vi "buildTestScenario.vi"(0 "TestScenarioFactory in":refnum<class "TestScenarioFactory.lvclass">, 5 "Log":refnum<class "ITestLog.lvclass">, 7 "Test Scenario":T1, 11 "error in (no error)":errorcluster) -> (4 "TestScenarioFactory out":refnum<class "TestScenarioFactory.lvclass">, 6 "ITestScenario.lvclass":refnum<class "ITestScenario.lvclass">, 15 "error out":errorcluster)   [LabVIEW 2015, in "TestScenarioFactory.lvclass"]
uses:
  TestScenarioFactory.lvclass
  Typedefs/TestScenarioTypes.ctl
  TestScenario/ITestScenario/ITestScenario.lvclass
  TestLog/ITestLog/ITestLog.lvclass
  TestScenario/Not Implemented Test/NotImplementedTest.lvclass
  TestScenario/Constant Analog Output Voltage Test/Constant Analog Output Voltage Test.lvclass
  TestScenarioFactory.lvclass/TestScenarioFactory.ctl
  TestScenario/Constant Current Output Test/Constant Current Output Test.lvclass
  TestScenario/Set DAC Test/Set ILC Test.lvclass
  ConfigureILCStrategy/ConfigureILCDCADAC1Strategy/ConfigureILCDCADAC1Strategy.lvclass
  ConfigureILCStrategy/ConfigureILCDCADAC2Strategy/ConfigureILCDCADAC2Strategy.lvclass
  ConfigureILCStrategy/ConfigureILCSSRStrategy/ConfigureILCSSRStrategy/ConfigureILCSSRStrategy.lvclass
  ConfigureILCStrategy/ConfigureILCDCAOutputStrategy/ConfigureILCDCAOutputStrategy.lvclass
  TestScenario/Verify ILC Test/Verify ILC Test.lvclass
  ReadILCStrategy/ReadILCDCAOutputStrategy/ReadILCDCAOutputStrategy.lvclass
  ConfigureILCStrategy/ConfigureILCDCAPressureStrategy/ConfigureILCDCAPressureStrategy.lvclass
  ReadILCStrategy/ReadILCDCAPowerFailStrategy/ReadILCDCAPowerFailStrategy.lvclass
  ReadILCStrategy/ReadILCDCAAmp1FailStrategy/ReadILCDCAAmp1FailStrategy.lvclass
  ReadILCStrategy/ReadILCDCAAmp2FailStrategy/ReadILCDCAAmp2FailStrategy.lvclass
  TestScenario/Test Pressure/Test Pressure.lvclass
  ConfigureILCStrategy/ConfigureILCDAC1Strategy/ConfigureILCDAC1Strategy.lvclass
  ReadILCStrategy/ReadILCDCAPressure1Strategy/ReadILCDCAPressure1Strategy.lvclass
  ConfigureILCStrategy/ConfigureILCDAC2Strategy/ConfigureILCDAC2Strategy.lvclass
  ReadILCStrategy/ReadILCDCAPressure2Strategy/ReadILCDCAPressure2Strategy.lvclass
  ConfigureILCStrategy/ConfigureILCDAC3Strategy/ConfigureILCDAC3Strategy.lvclass
  ReadILCStrategy/ReadILCDCAPressure3Strategy/ReadILCDCAPressure3Strategy.lvclass
  ConfigureILCStrategy/ConfigureILCDAC4Strategy/ConfigureILCDAC4Strategy.lvclass
  ReadILCStrategy/ReadILCDCAPressure4Strategy/ReadILCDCAPressure4Strategy.lvclass
  TestScenario/Current Linear Test/Current Linear Test.lvclass
  Typedefs/ILCBTTypedefs.lvlib
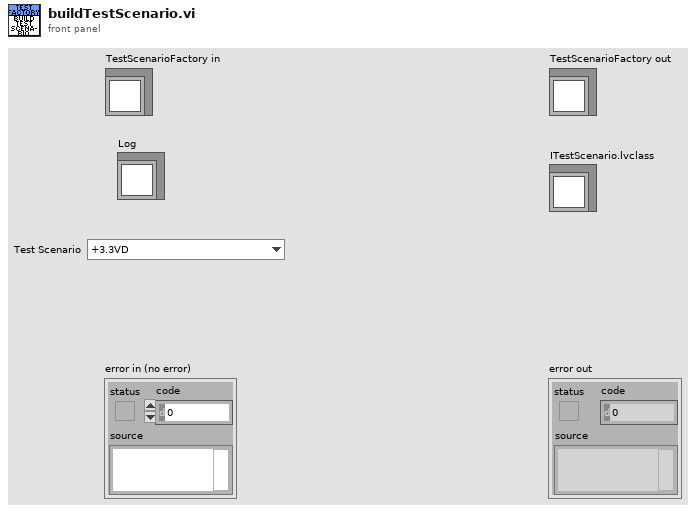
[diagram p1: front panel]
types:
  T1 = typedef "ILCBTTypedefs.lvlib/TestScenarioTypes.ctl" = enum16{"+3.3VD", "+5.1V", "+24V", "RELVALV1", "RELVALV2", "Verify DAC_A = -1.00A", "Verify DAC_A = -0.75A", "Verify DAC_A = -0.50A", "Verify DAC_A = -0.25A", "Verify DAC_A = 0.00A", "Verify DAC_A = 0.25A", "Verify DAC_A = 0.50A", "Verify DAC_A = 0.75A", "Verify DAC_A = 1.00A", "Verify DAC_B = -1.00A", "Verify DAC_B = -0.75A", "Verify DAC_B = -0.50A", "Verify DAC_B = -0.25A", "Verify DAC_B = 0.00A", "Verify DAC_B = 0.25A", "Verify DAC_B = 0.50A", "Verify DAC_B = 0.75A", "Verify DAC_B = 1.00A", "Set DAC_A = -1.00A", "Set DAC_A = -0.75A", "Set DAC_A = -0.50A", "Set DAC_A = -0.25A", "Set DAC_A = 0.00A", "Set DAC_A = 0.25A", "Set DAC_A = 0.50A", "Set DAC_A = 0.75A", "Set DAC_A = 1.00A", "Set DAC_B = -1.00A", "Set DAC_B = -0.75A", "Set DAC_B = -0.50A", "Set DAC_B = -0.25A", "Set DAC_B = 0.00A", "Set DAC_B = 0.25A", "Set DAC_B = 0.50A", "Set DAC_B = 0.75A", "Set DAC_B = 1.00A", "Set MTR_PWR = On", "Set MTR_PWR = Off", "Set OUTPUT = On", "Set OUTPUT = Off", "Verify OUTPUT = On", "Verify OUTPUT = Off", "Verify POWER = Ok", "Verify POWER = Fail", "Verify AMP1 = Ok", "Verify AMP1 = Fail", "Verify AMP2 = Ok", "Verify AMP2 = Fail", "P1 0%", "P1 25%", "P1 50%", "P1 75%", "P1 100%", "P2 0%", "P2 25%", "P2 50%", "P2 75%", "P2 100%", "P3 0%", "P3 25%", "P3 50%", "P3 75%", "P3 100%", "P4 0%", "P4 25%", "P4 50%", "P4 75%", "P4 100%", "DCA 1 Linearity", "DCA 2 Linearity"}
  T2 = typedef "ILCBTTypedefs.lvlib/Pressure Test.ctl" = cluster{"Command":u16, "Expected":u16, "Tolerance":u16}
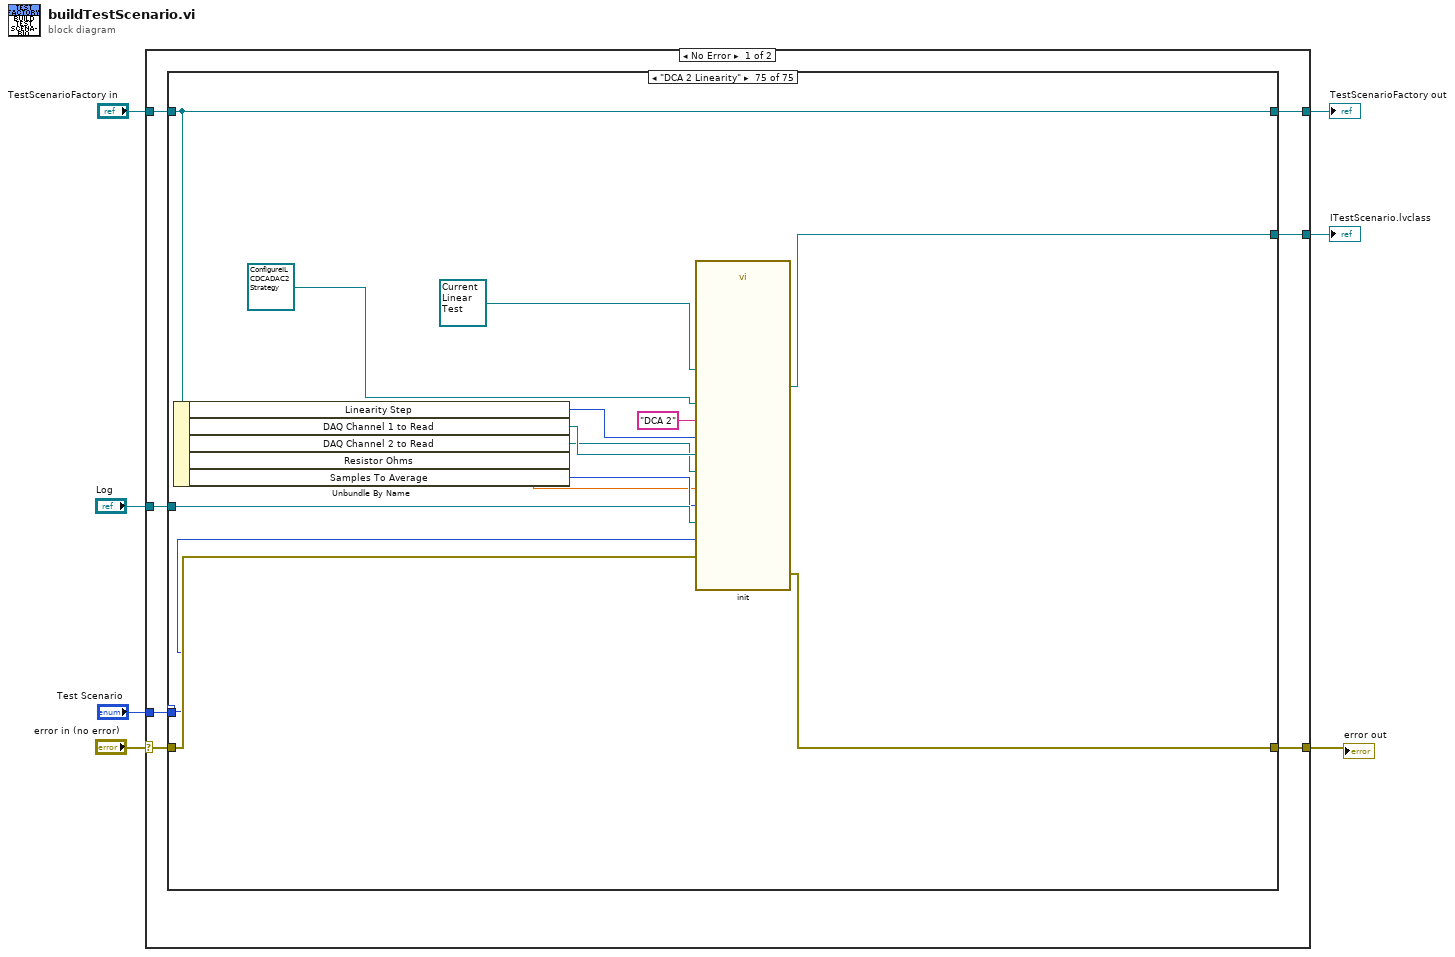
[diagram p0: block diagram]
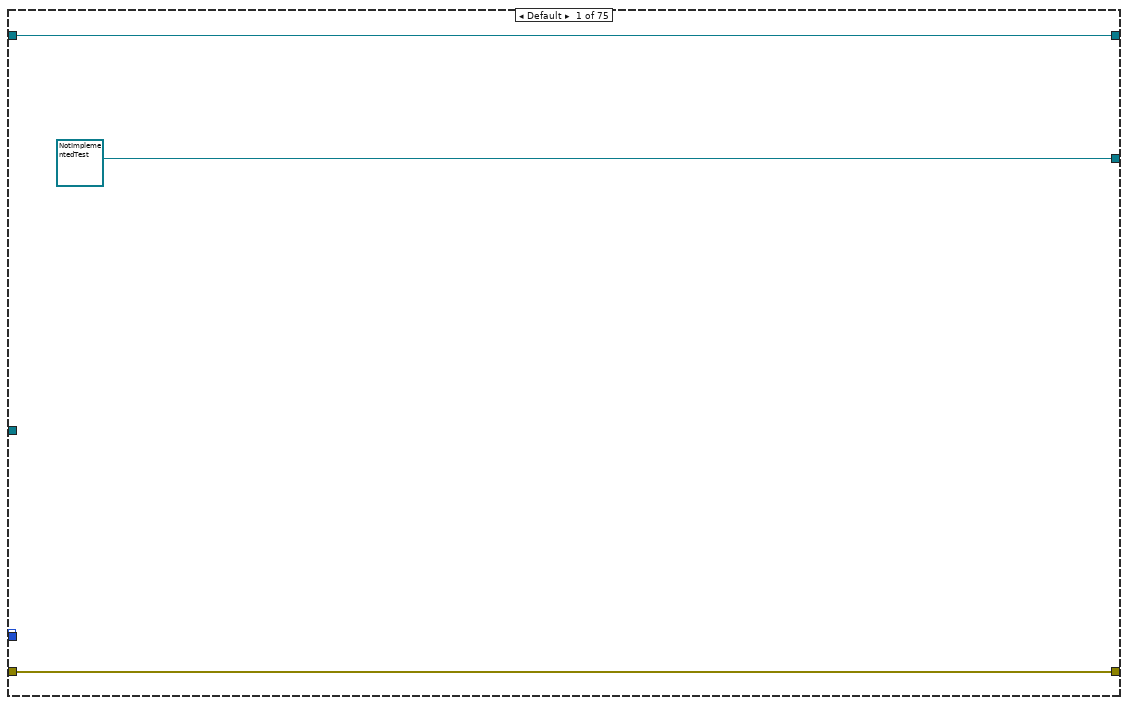
[diagram p2: hidden frame]
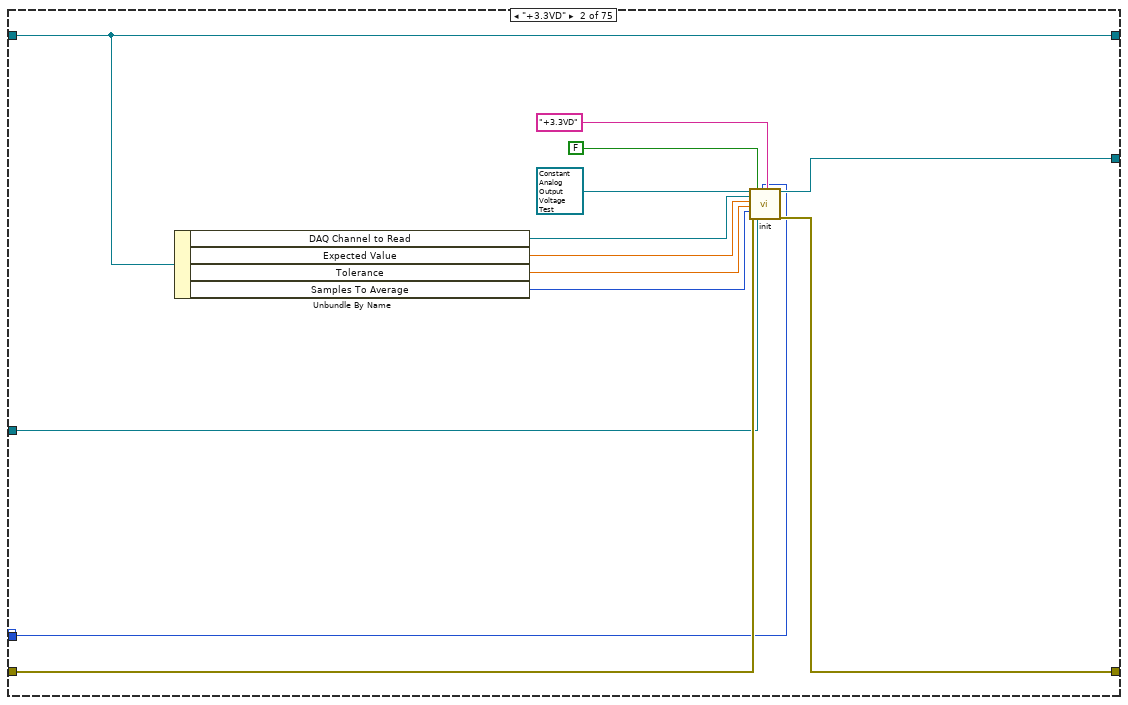
[diagram p3: hidden frame]
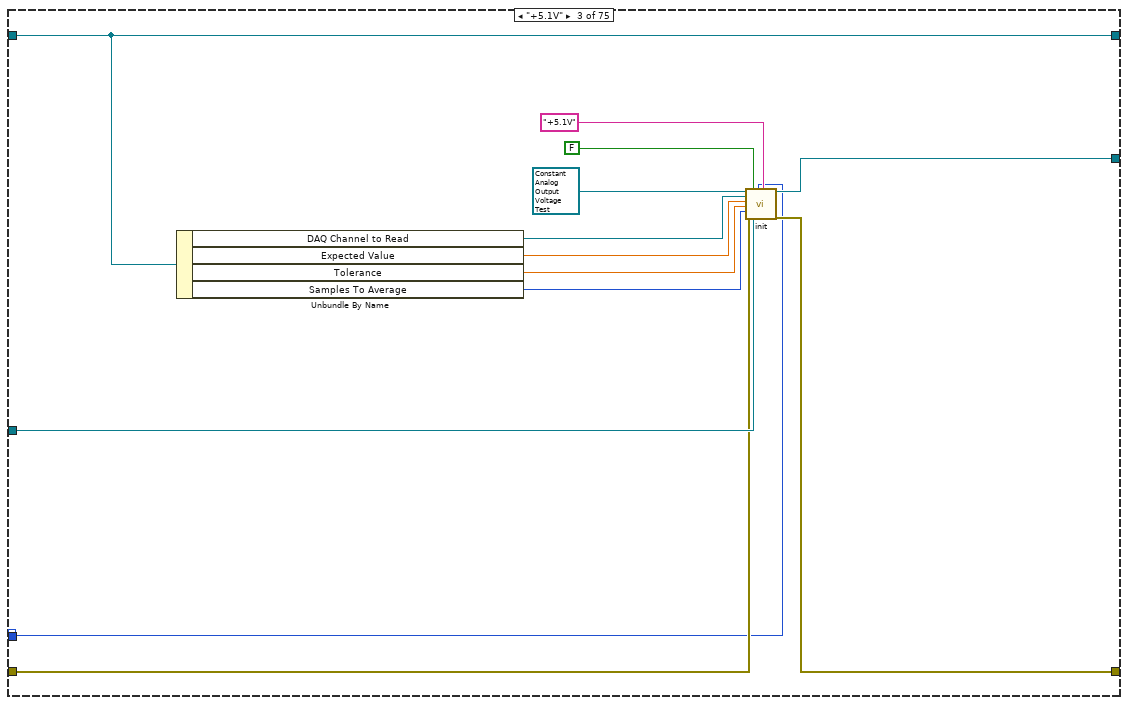
[diagram p4: hidden frame]
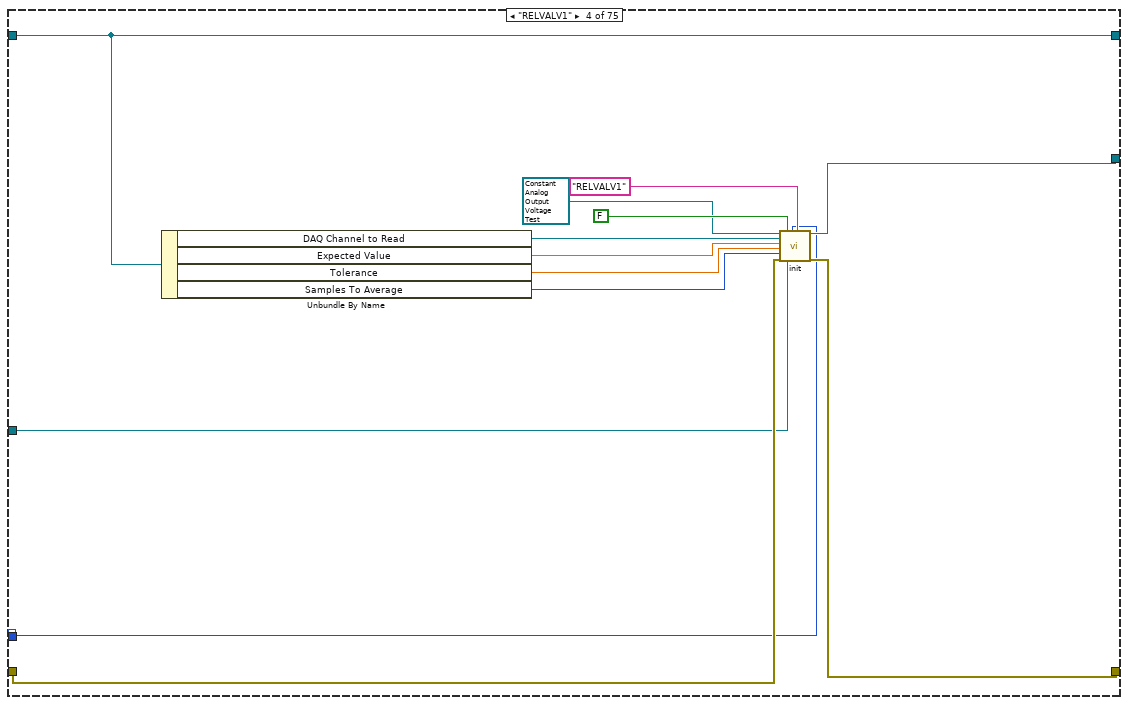
[diagram p5: hidden frame]
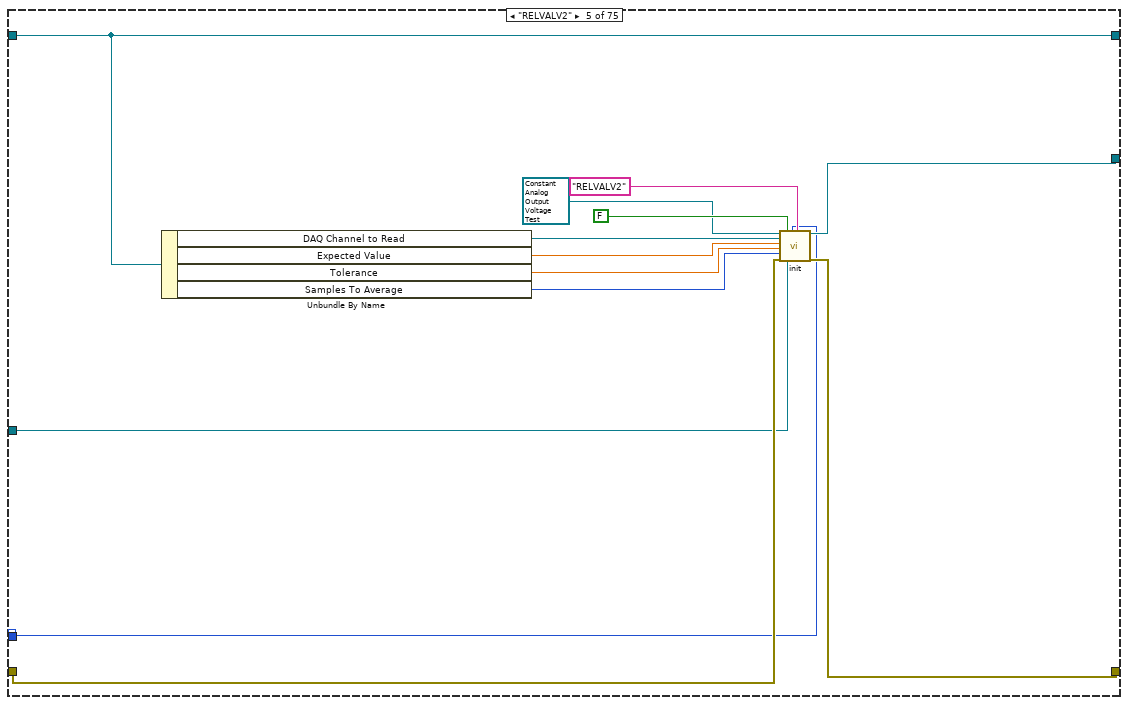
[diagram p6: hidden frame]
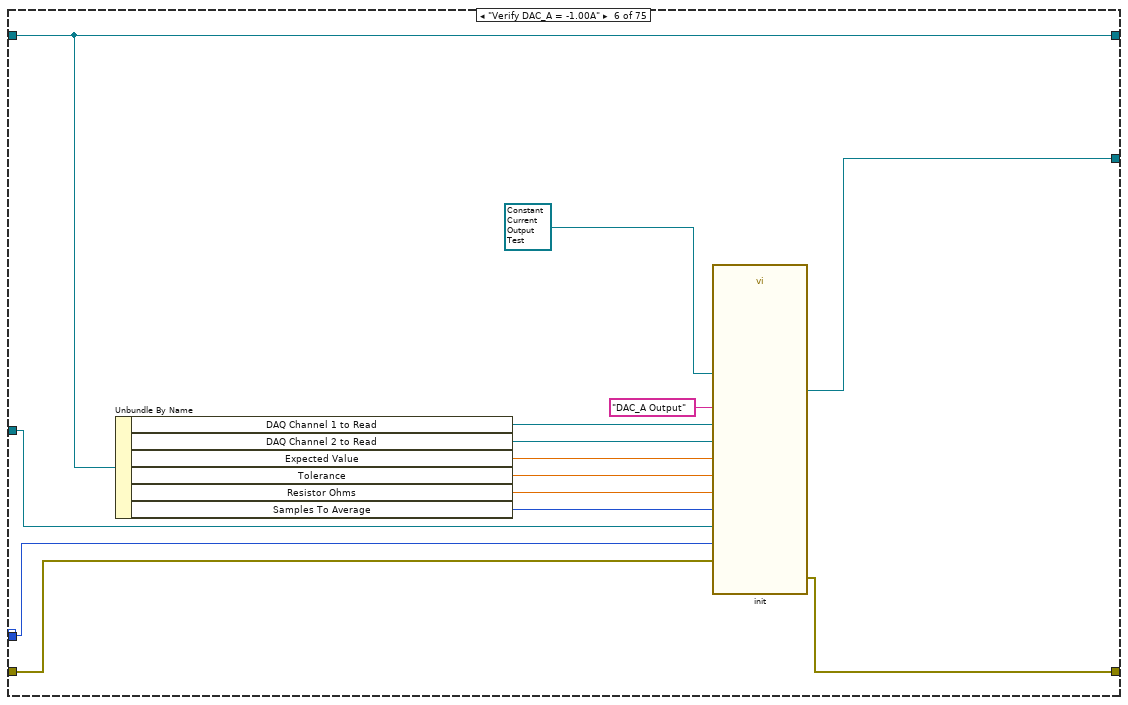
[diagram p7: hidden frame]
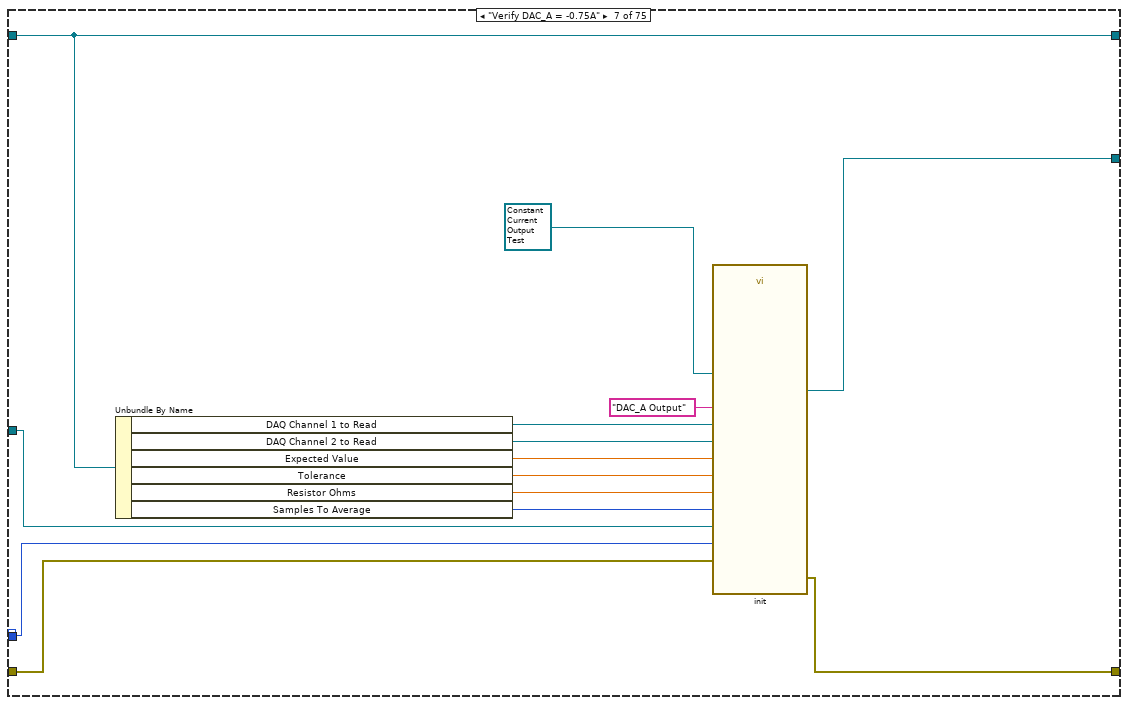
[diagram p8: hidden frame]
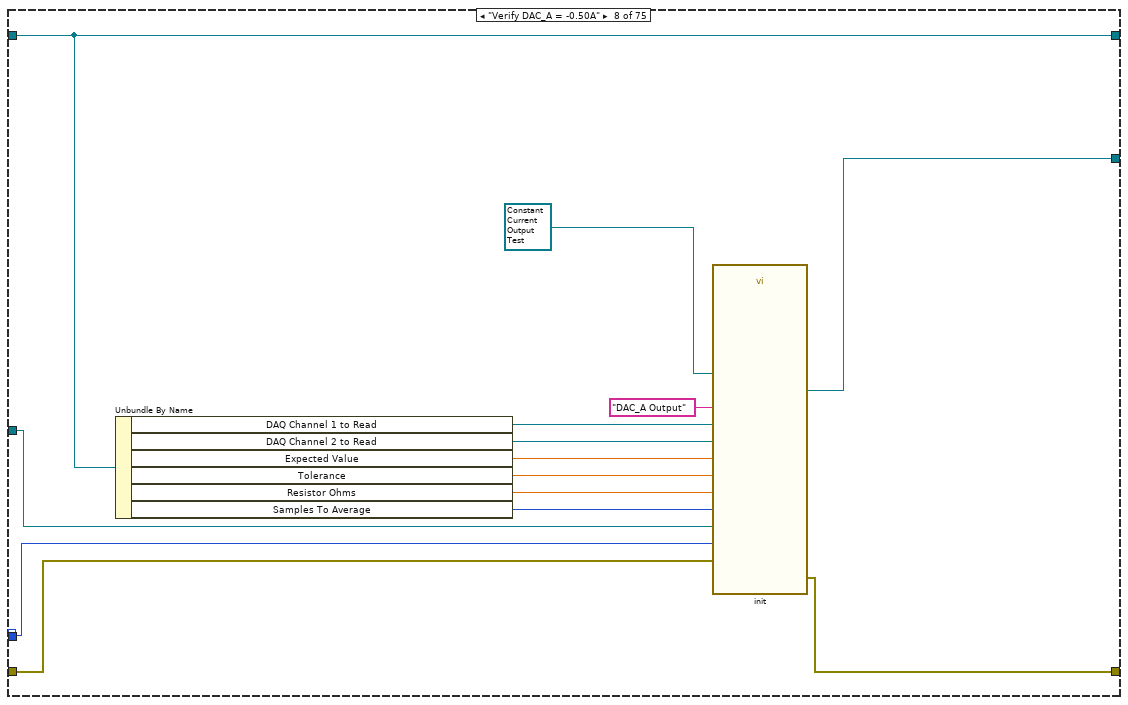
[diagram p9: hidden frame]
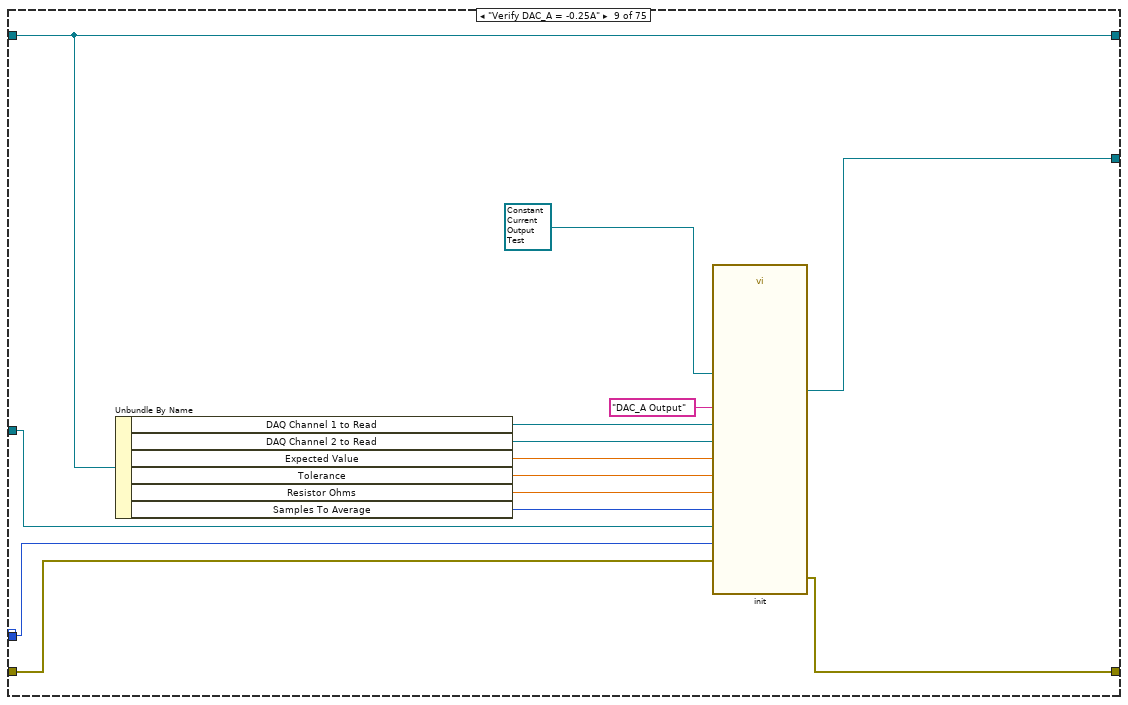
[diagram p10: hidden frame]
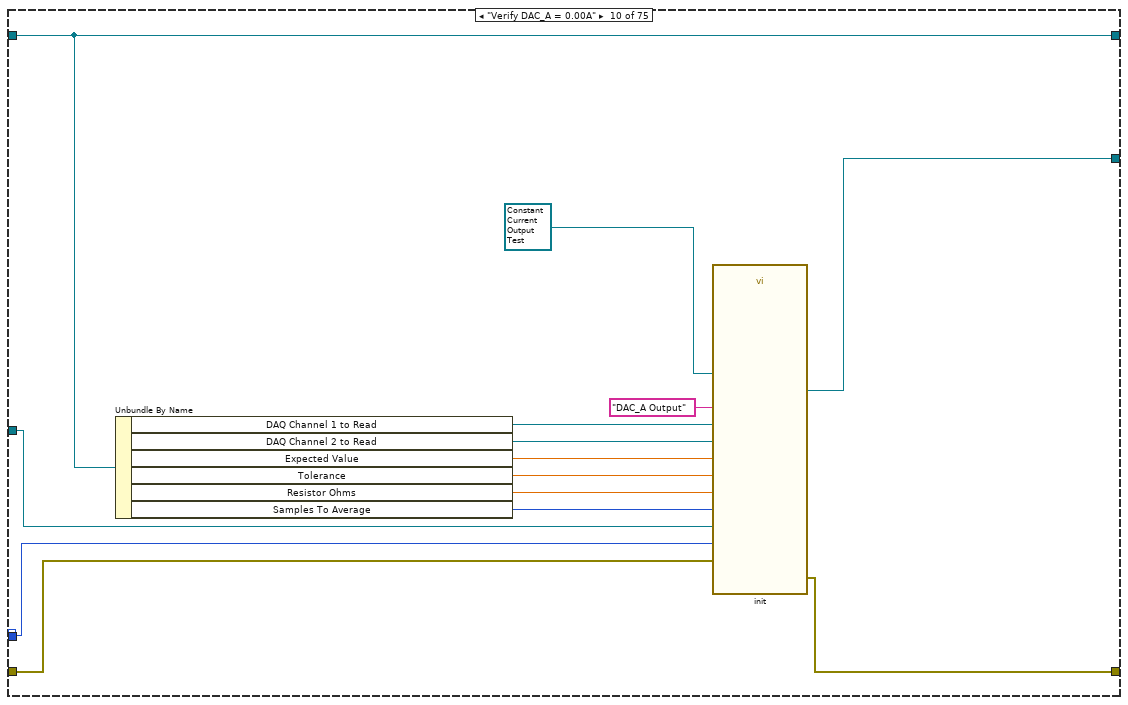
[diagram p11: hidden frame]
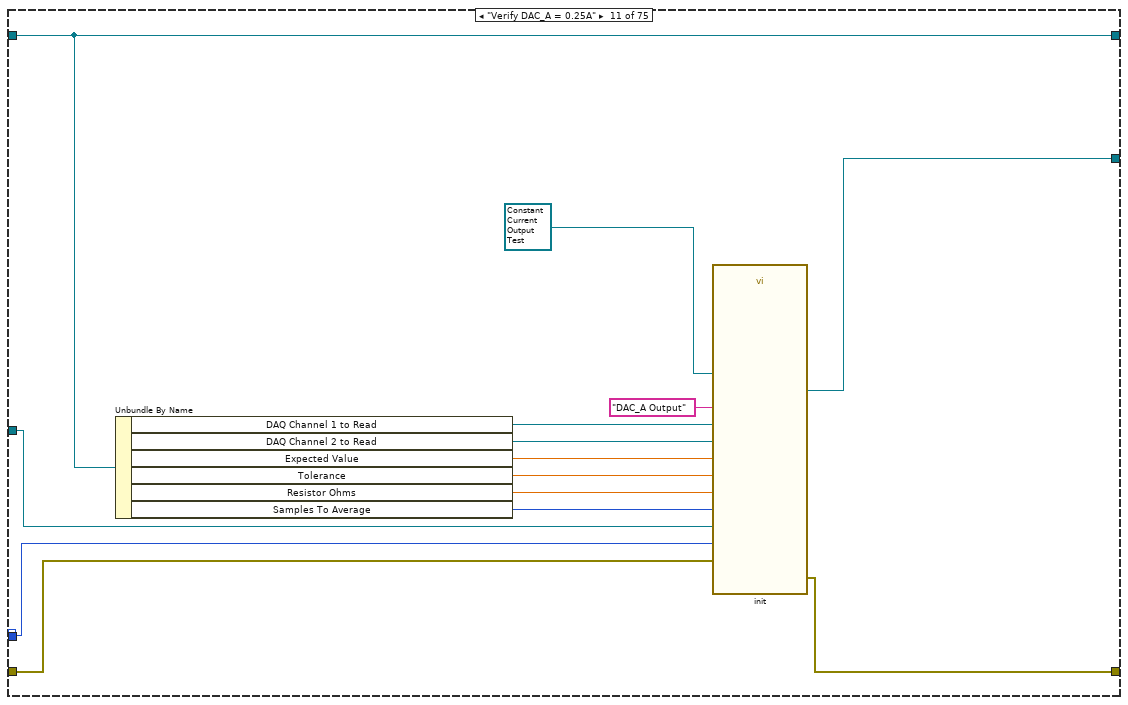
[diagram p12: hidden frame]
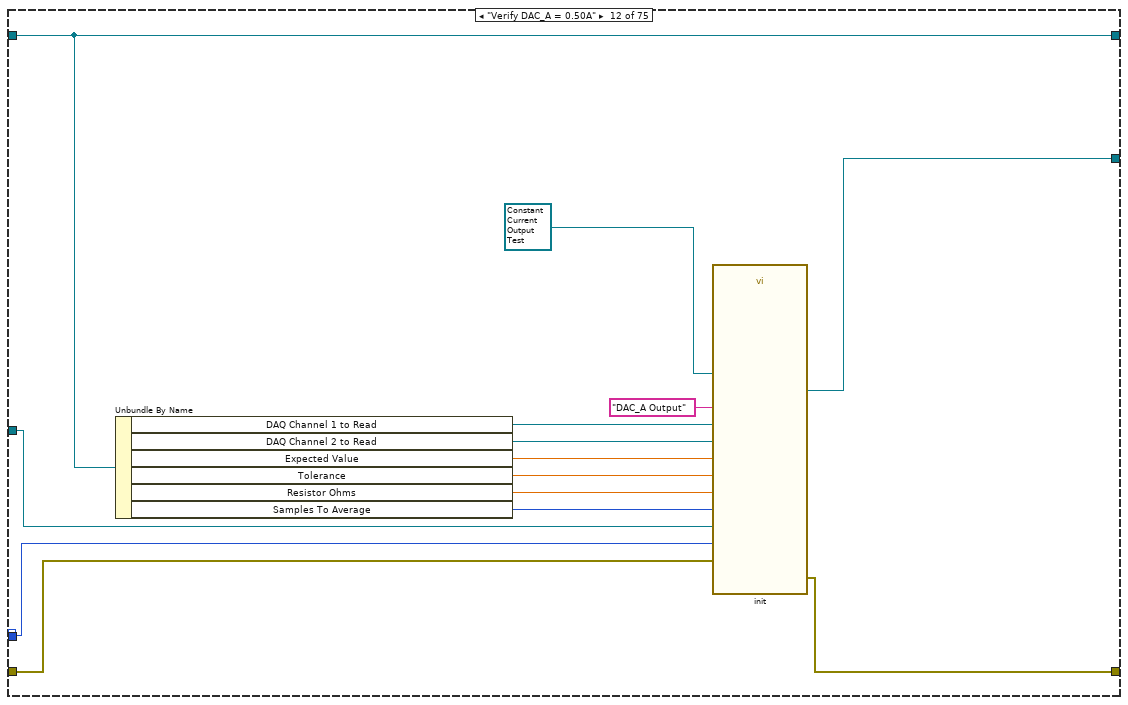
[diagram p13: hidden frame]
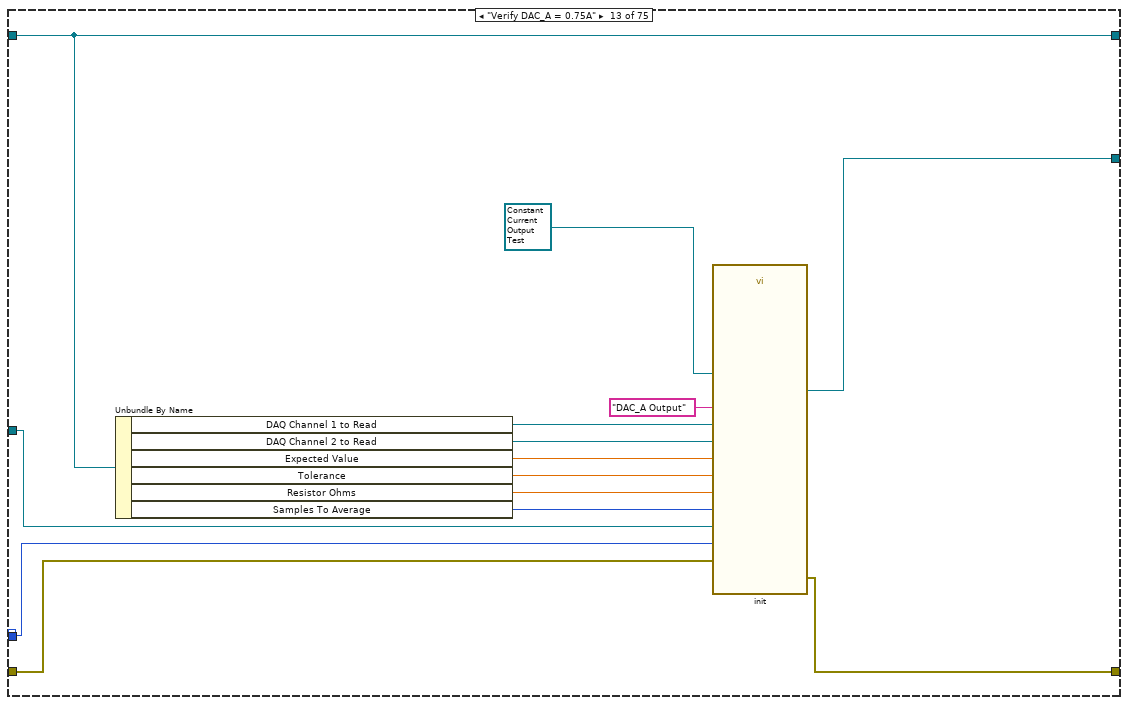
[diagram p14: hidden frame]
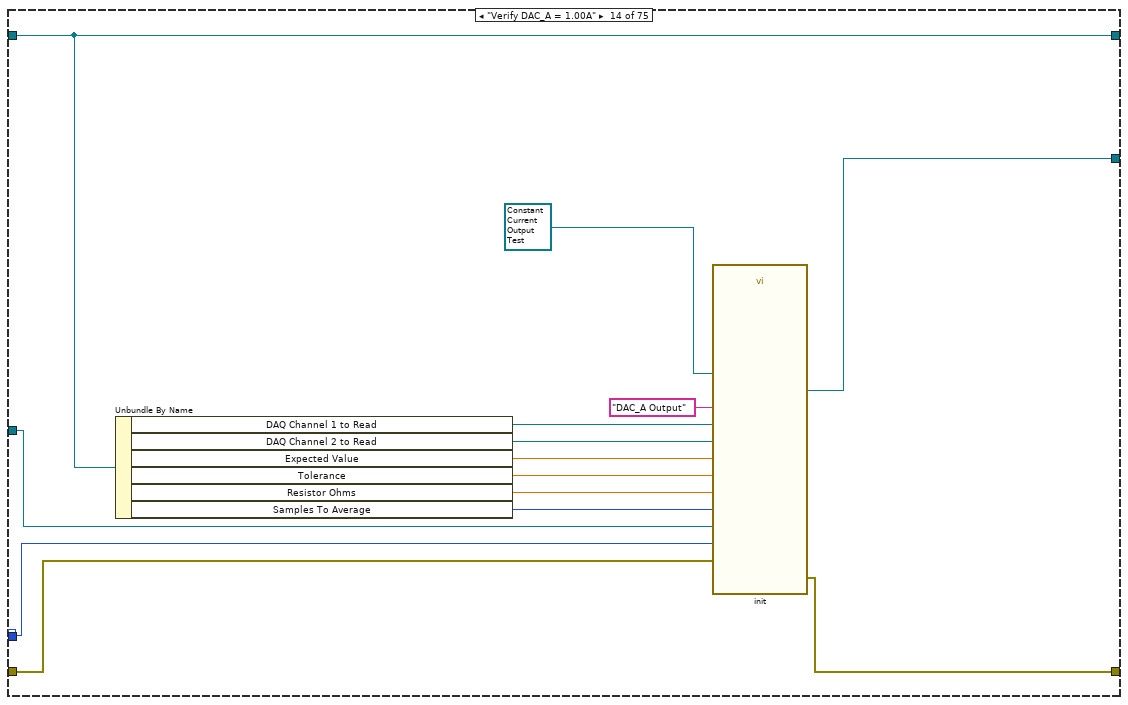
[diagram p15: hidden frame]
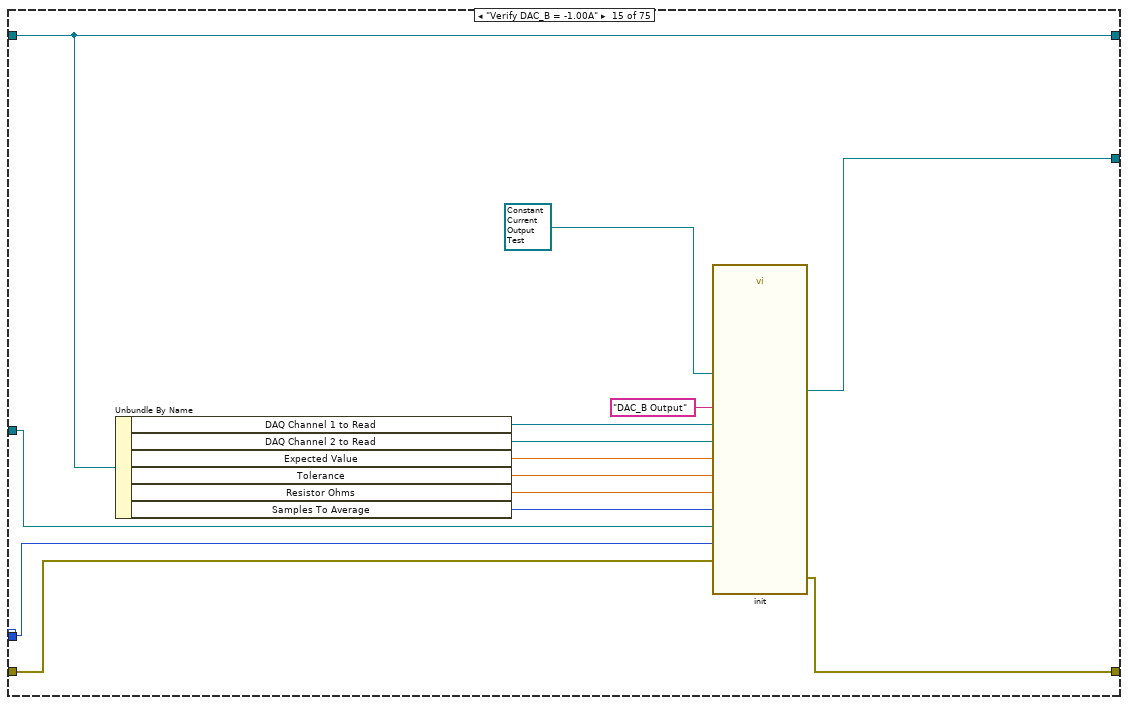
[diagram p16: hidden frame]
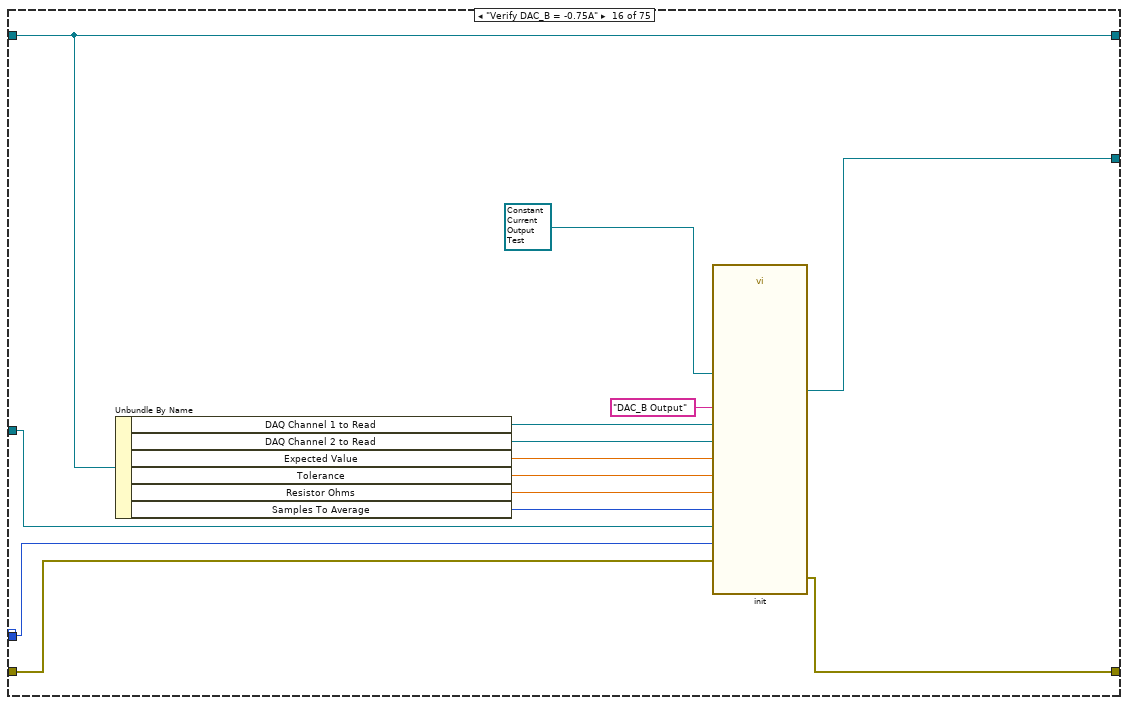
[diagram p17: hidden frame]
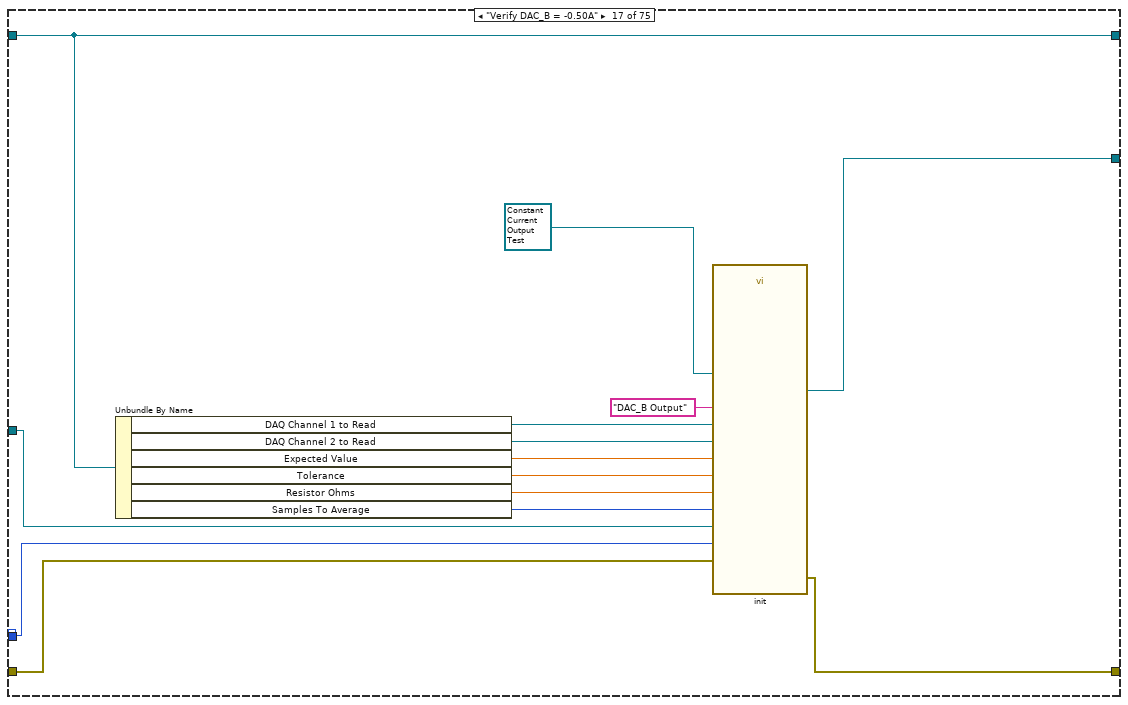
[diagram p18: hidden frame]
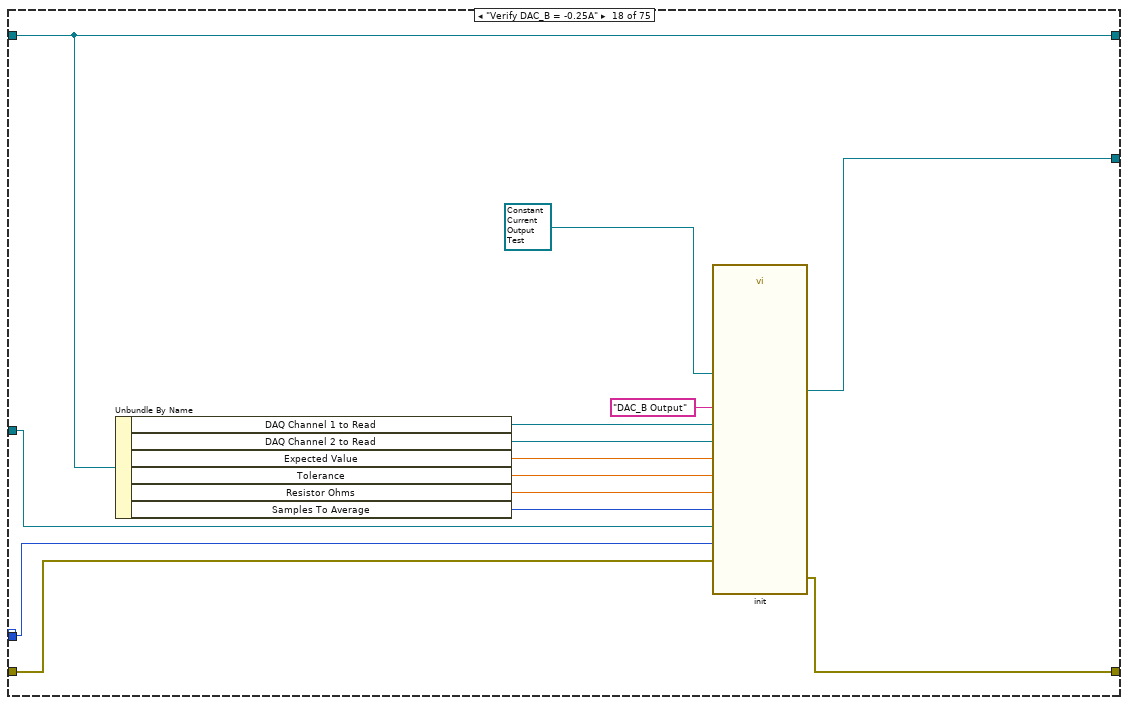
[diagram p19: hidden frame]
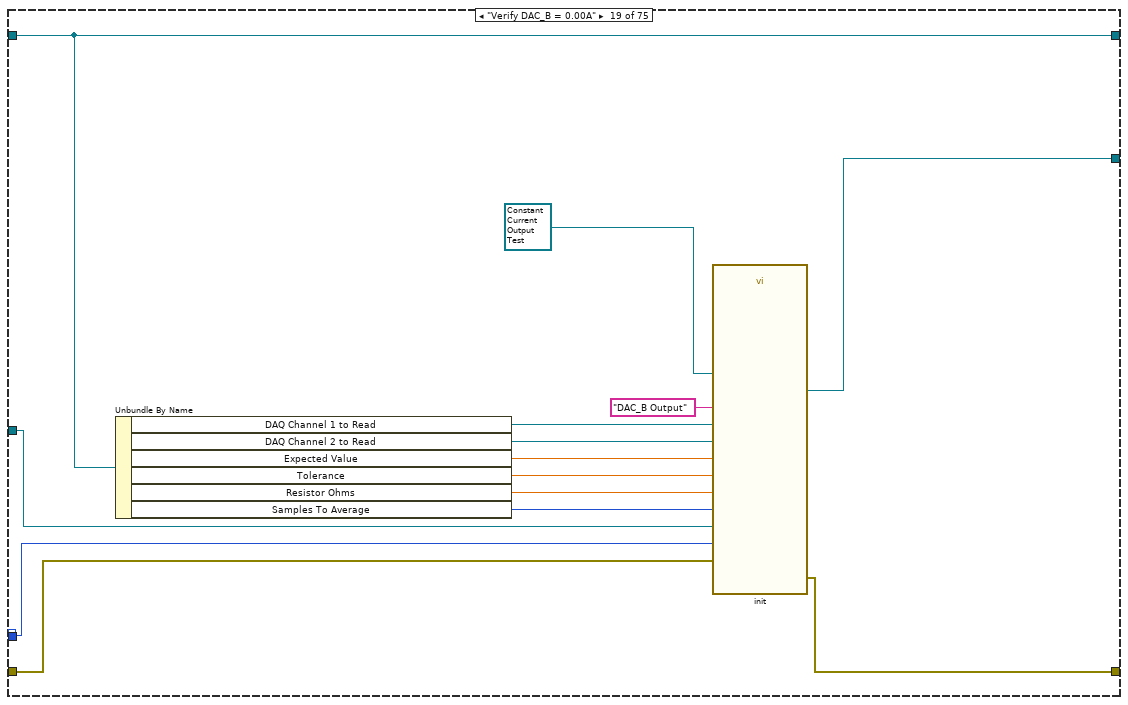
[diagram p20: hidden frame]
diagram:
  n1 = case shown="No Error" "error in (no error)" {
    selector: "error in (no error)" -> [w13 w948]
    tunnel: "Test Scenario" -> [w8 _]
    tunnel: "TestScenarioFactory in" -> [w14 w947]
    tunnel: [w12 w948] -> w3
    tunnel: [w9 w947] -> w5
    tunnel: "Log" -> [w10 _]
    tunnel: [w11 refnum<class "ITestScenario.lvclass"> refnum ("ITestScenario.lvclass")] -> w1
    frame No Error {
      n2 = case shown="\"DCA 2 Linearity\"" w8 {
        selector: w8 -> [_ w18 w31 w44 w57 w79 w93 w107 w121 w135 w149 w163 w177 w191 w205 w219 w233 w247 w261 w275 w289 w303 w317 w329 w339 w349 w359 w369 w379 w389 w399 w409 w419 w429 w439 w449 w459 w469 w479 w489 w499 w509 w519 w529 w539 w548 w560 w572 w584 w596 w608 w620 w632 w647 w661 w675 w689 w703 w717 w731 w745 w759 w773 w787 w801 w815 w829 w843 w857 w871 w885 w899 w913 w928 w942]
        tunnel: w14 -> [w17 w30 w34 w45 w58 w78 w92 w106 w120 w134 w148 w162 w176 w190 w204 w218 w232 w246 w260 w274 w288 w302 w316 w324 w334 w344 w354 w364 w374 w384 w394 w404 w415 w425 w435 w445 w455 w465 w475 w485 w495 w505 w515 w525 w535 w553 w565 w577 w589 w601 w613 w625 w637 w642 w656 w670 w684 w698 w714 w728 w742 w756 w770 w784 w798 w812 w826 w840 w854 w868 w882 w896 w910 w918 w933]
        tunnel: w13 -> [w16 w27 w35 w48 w61 w83 w97 w111 w125 w139 w153 w167 w181 w195 w209 w223 w237 w251 w265 w279 w293 w307 w321 w328 w338 w348 w358 w368 w378 w388 w398 w408 w418 w428 w438 w448 w458 w468 w478 w488 w498 w508 w518 w528 w538 w549 w561 w573 w585 w597 w609 w621 w633 w649 w663 w677 w691 w705 w719 w733 w747 w761 w775 w789 w803 w817 w831 w845 w859 w873 w887 w901 w915 w929 w943]
        tunnel: [w16 w19 w32 w49 w62 w82 w96 w110 w124 w138 w152 w166 w180 w194 w208 w222 w236 w250 w264 w278 w292 w306 w320 w327 w337 w347 w357 w367 w377 w387 w397 w407 w417 w427 w437 w447 w457 w467 w477 w487 w497 w507 w517 w527 w537 w550 w562 w574 w586 w598 w610 w622 w634 w648 w662 w676 w690 w704 w718 w732 w746 w760 w774 w788 w802 w816 w830 w844 w858 w872 w886 w900 w914 w927 w941] -> w12
        tunnel: [refnum<class "NotImplementedTest.lvclass"> refnum ("NotImplementedTest.lvclass") w28 w33 w46 w59 w81 w95 w109 w123 w137 w151 w165 w179 w193 w207 w221 w235 w249 w263 w277 w291 w305 w319 w331 w341 w351 w361 w371 w381 w391 w401 w411 w421 w431 w441 w451 w461 w471 w481 w491 w501 w511 w521 w531 w541 w551 w563 w575 w587 w599 w611 w623 w635 w650 w664 w678 w692 w706 w720 w734 w748 w762 w776 w790 w804 w818 w832 w846 w860 w874 w888 w902 w916 w930 w944] -> w11
        tunnel: w10 -> [_ w26 w36 w47 w60 w80 w94 w108 w122 w136 w150 w164 w178 w192 w206 w220 w234 w248 w262 w276 w290 w304 w318 w326 w336 w346 w356 w366 w376 w386 w396 w406 w416 w426 w436 w446 w456 w466 w476 w486 w496 w506 w516 w526 w536 w547 w559 w571 w583 w595 w607 w619 w631 w646 w660 w674 w688 w702 w716 w730 w744 w758 w772 w786 w800 w814 w828 w842 w856 w870 w884 w898 w912 w926 w940]
        tunnel: [w17 w30 w34 w45 w58 w78 w92 w106 w120 w134 w148 w162 w176 w190 w204 w218 w232 w246 w260 w274 w288 w302 w316 w324 w334 w344 w354 w364 w374 w384 w394 w404 w415 w425 w435 w445 w455 w465 w475 w485 w495 w505 w515 w525 w535 w553 w565 w577 w589 w601 w613 w625 w637 w642 w656 w670 w684 w698 w714 w728 w742 w756 w770 w784 w798 w812 w826 w840 w854 w868 w882 w896 w910 w918 w933] -> w9
        tunnel: w8 -> [_ _ _ _ _ _ _ _ _ _ _ _ _ _ _ _ _ _ _ _ _ _ _ _ _ _ _ _ _ _ _ _ _ _ _ _ _ _ _ _ _ _ _ _ _ _ _ _ _ _ _ _ _ _ _ _ _ _ _ _ _ _ _ _ _ _ _ _ _ _ _ _ _ _ _]
        frame Default {
        }
        frame "+3.3VD" {
          n3 = Unbundle By Name(w30) -> ("DAQ Channel to Read"=w22:refnum<k21>, "Expected Value"=w23:dbl, "Tolerance"=w24:dbl, "Samples To Average"=w25:i32)
          n4 = call "init.vi"("Constant Analog Output Voltage Test in"=refnum<class "Constant Analog Output Voltage Test.lvclass"> refnum ("Constant Analog Input Voltage Test.lvclass"), "DAQ Channel"=w22, "Expected Value"=w23, "Tolerance"=w24, "Samples To Average"=w25, "error in (no error)"=w27, "MustPass?"=FALSE, "Log"=w26, "Test Scenario"=w18, "Signal Name"="+3.3VD") -> ("Constant Analog Output Voltage Test  out"=w28:refnum<class "Constant Analog Output Voltage Test.lvclass">, "error out"=w19:errorcluster)  [unwired: 8 in]
        }
        frame "+5.1V" {
          n5 = Unbundle By Name(w34) -> ("DAQ Channel to Read"=w39:refnum<k21>, "Expected Value"=w40:dbl, "Tolerance"=w41:dbl, "Samples To Average"=w42:i32)
          n6 = call "init.vi"("Constant Analog Output Voltage Test in"=refnum<class "Constant Analog Output Voltage Test.lvclass"> refnum ("Constant Analog Input Voltage Test.lvclass"), "DAQ Channel"=w39, "Expected Value"=w40, "Tolerance"=w41, "Samples To Average"=w42, "error in (no error)"=w35, "MustPass?"=FALSE, "Log"=w36, "Test Scenario"=w31, "Signal Name"="+5.1V") -> ("Constant Analog Output Voltage Test  out"=w33:refnum<class "Constant Analog Output Voltage Test.lvclass">, "error out"=w32:errorcluster)  [unwired: 8 in]
        }
        frame "RELVALV1" {
          n7 = Unbundle By Name(w45) -> ("DAQ Channel to Read"=w54:refnum<k21>, "Expected Value"=w53:dbl, "Tolerance"=w52:dbl, "Samples To Average"=w51:i32)
          n8 = call "init.vi"("Constant Analog Output Voltage Test in"=refnum<class "Constant Analog Output Voltage Test.lvclass"> refnum ("Constant Analog Input Voltage Test.lvclass"), "DAQ Channel"=w54, "Expected Value"=w53, "Tolerance"=w52, "Samples To Average"=w51, "error in (no error)"=w48, "MustPass?"=FALSE, "Log"=w47, "Test Scenario"=w44, "Signal Name"="RELVALV1") -> ("Constant Analog Output Voltage Test  out"=w46:refnum<class "Constant Analog Output Voltage Test.lvclass">, "error out"=w49:errorcluster)  [unwired: 8 in]
        }
        frame "RELVALV2" {
          n9 = Unbundle By Name(w58) -> ("DAQ Channel to Read"=w67:refnum<k21>, "Expected Value"=w66:dbl, "Tolerance"=w65:dbl, "Samples To Average"=w64:i32)
          n10 = call "init.vi"("Constant Analog Output Voltage Test in"=refnum<class "Constant Analog Output Voltage Test.lvclass"> refnum ("Constant Analog Input Voltage Test.lvclass"), "DAQ Channel"=w67, "Expected Value"=w66, "Tolerance"=w65, "Samples To Average"=w64, "error in (no error)"=w61, "MustPass?"=FALSE, "Log"=w60, "Test Scenario"=w57, "Signal Name"="RELVALV2") -> ("Constant Analog Output Voltage Test  out"=w59:refnum<class "Constant Analog Output Voltage Test.lvclass">, "error out"=w62:errorcluster)  [unwired: 8 in]
        }
        frame "Verify DAC_A = -1.00A" {
          n11 = Unbundle By Name(w78) -> ("DAQ Channel 1 to Read"=w72:refnum<k21>, "DAQ Channel 2 to Read"=w73:refnum<k21>, "Expected Value"=w74:dbl, "Tolerance"=w75:dbl, "Resistor Ohms"=w76:dbl, "Samples To Average"=w77:i32)
          n12 = call "init.vi"("Constant Analog Output Voltage Test in"=refnum<class "Constant Current Output Test.lvclass"> refnum ("Constant Current Output Test.lvclass"), "DAQ Channel 1"=w72, "Expected Value"=w74, "Tolerance"=w75, "Samples To Average"=w77, "error in (no error)"=w83, "DAQ Channel 2"=w73, "Log"=w80, "Test Scenario"=w79, "Resistance"=w76, "Signal Name"="DAC_A Output") -> ("Constant Analog Output Voltage Test  out"=w81:refnum<class "Constant Current Output Test.lvclass">, "error out"=w82:errorcluster)  [unwired: 7 in]
        }
        frame "Verify DAC_A = -0.75A" {
          n13 = Unbundle By Name(w92) -> ("DAQ Channel 1 to Read"=w86:refnum<k21>, "DAQ Channel 2 to Read"=w87:refnum<k21>, "Expected Value"=w88:dbl, "Tolerance"=w89:dbl, "Resistor Ohms"=w90:dbl, "Samples To Average"=w91:i32)
          n14 = call "init.vi"("Constant Analog Output Voltage Test in"=refnum<class "Constant Current Output Test.lvclass"> refnum ("Constant Current Output Test.lvclass"), "DAQ Channel 1"=w86, "Expected Value"=w88, "Tolerance"=w89, "Samples To Average"=w91, "error in (no error)"=w97, "DAQ Channel 2"=w87, "Log"=w94, "Test Scenario"=w93, "Resistance"=w90, "Signal Name"="DAC_A Output") -> ("Constant Analog Output Voltage Test  out"=w95:refnum<class "Constant Current Output Test.lvclass">, "error out"=w96:errorcluster)  [unwired: 7 in]
        }
        frame "Verify DAC_A = -0.50A" {
          n15 = Unbundle By Name(w106) -> ("DAQ Channel 1 to Read"=w100:refnum<k21>, "DAQ Channel 2 to Read"=w101:refnum<k21>, "Expected Value"=w102:dbl, "Tolerance"=w103:dbl, "Resistor Ohms"=w104:dbl, "Samples To Average"=w105:i32)
          n16 = call "init.vi"("Constant Analog Output Voltage Test in"=refnum<class "Constant Current Output Test.lvclass"> refnum ("Constant Current Output Test.lvclass"), "DAQ Channel 1"=w100, "Expected Value"=w102, "Tolerance"=w103, "Samples To Average"=w105, "error in (no error)"=w111, "DAQ Channel 2"=w101, "Log"=w108, "Test Scenario"=w107, "Resistance"=w104, "Signal Name"="DAC_A Output") -> ("Constant Analog Output Voltage Test  out"=w109:refnum<class "Constant Current Output Test.lvclass">, "error out"=w110:errorcluster)  [unwired: 7 in]
        }
        frame "Verify DAC_A = -0.25A" {
          n17 = Unbundle By Name(w120) -> ("DAQ Channel 1 to Read"=w114:refnum<k21>, "DAQ Channel 2 to Read"=w115:refnum<k21>, "Expected Value"=w116:dbl, "Tolerance"=w117:dbl, "Resistor Ohms"=w118:dbl, "Samples To Average"=w119:i32)
          n18 = call "init.vi"("Constant Analog Output Voltage Test in"=refnum<class "Constant Current Output Test.lvclass"> refnum ("Constant Current Output Test.lvclass"), "DAQ Channel 1"=w114, "Expected Value"=w116, "Tolerance"=w117, "Samples To Average"=w119, "error in (no error)"=w125, "DAQ Channel 2"=w115, "Log"=w122, "Test Scenario"=w121, "Resistance"=w118, "Signal Name"="DAC_A Output") -> ("Constant Analog Output Voltage Test  out"=w123:refnum<class "Constant Current Output Test.lvclass">, "error out"=w124:errorcluster)  [unwired: 7 in]
        }
        frame "Verify DAC_A = 0.00A" {
          n19 = Unbundle By Name(w134) -> ("DAQ Channel 1 to Read"=w128:refnum<k21>, "DAQ Channel 2 to Read"=w129:refnum<k21>, "Expected Value"=w130:dbl, "Tolerance"=w131:dbl, "Resistor Ohms"=w132:dbl, "Samples To Average"=w133:i32)
          n20 = call "init.vi"("Constant Analog Output Voltage Test in"=refnum<class "Constant Current Output Test.lvclass"> refnum ("Constant Current Output Test.lvclass"), "DAQ Channel 1"=w128, "Expected Value"=w130, "Tolerance"=w131, "Samples To Average"=w133, "error in (no error)"=w139, "DAQ Channel 2"=w129, "Log"=w136, "Test Scenario"=w135, "Resistance"=w132, "Signal Name"="DAC_A Output") -> ("Constant Analog Output Voltage Test  out"=w137:refnum<class "Constant Current Output Test.lvclass">, "error out"=w138:errorcluster)  [unwired: 7 in]
        }
        frame "Verify DAC_A = 0.25A" {
          n21 = Unbundle By Name(w148) -> ("DAQ Channel 1 to Read"=w142:refnum<k21>, "DAQ Channel 2 to Read"=w143:refnum<k21>, "Expected Value"=w144:dbl, "Tolerance"=w145:dbl, "Resistor Ohms"=w146:dbl, "Samples To Average"=w147:i32)
          n22 = call "init.vi"("Constant Analog Output Voltage Test in"=refnum<class "Constant Current Output Test.lvclass"> refnum ("Constant Current Output Test.lvclass"), "DAQ Channel 1"=w142, "Expected Value"=w144, "Tolerance"=w145, "Samples To Average"=w147, "error in (no error)"=w153, "DAQ Channel 2"=w143, "Log"=w150, "Test Scenario"=w149, "Resistance"=w146, "Signal Name"="DAC_A Output") -> ("Constant Analog Output Voltage Test  out"=w151:refnum<class "Constant Current Output Test.lvclass">, "error out"=w152:errorcluster)  [unwired: 7 in]
        }
        frame "Verify DAC_A = 0.50A" {
          n23 = Unbundle By Name(w162) -> ("DAQ Channel 1 to Read"=w156:refnum<k21>, "DAQ Channel 2 to Read"=w157:refnum<k21>, "Expected Value"=w158:dbl, "Tolerance"=w159:dbl, "Resistor Ohms"=w160:dbl, "Samples To Average"=w161:i32)
          n24 = call "init.vi"("Constant Analog Output Voltage Test in"=refnum<class "Constant Current Output Test.lvclass"> refnum ("Constant Current Output Test.lvclass"), "DAQ Channel 1"=w156, "Expected Value"=w158, "Tolerance"=w159, "Samples To Average"=w161, "error in (no error)"=w167, "DAQ Channel 2"=w157, "Log"=w164, "Test Scenario"=w163, "Resistance"=w160, "Signal Name"="DAC_A Output") -> ("Constant Analog Output Voltage Test  out"=w165:refnum<class "Constant Current Output Test.lvclass">, "error out"=w166:errorcluster)  [unwired: 7 in]
        }
        frame "Verify DAC_A = 0.75A" {
          n25 = Unbundle By Name(w176) -> ("DAQ Channel 1 to Read"=w170:refnum<k21>, "DAQ Channel 2 to Read"=w171:refnum<k21>, "Expected Value"=w172:dbl, "Tolerance"=w173:dbl, "Resistor Ohms"=w174:dbl, "Samples To Average"=w175:i32)
          n26 = call "init.vi"("Constant Analog Output Voltage Test in"=refnum<class "Constant Current Output Test.lvclass"> refnum ("Constant Current Output Test.lvclass"), "DAQ Channel 1"=w170, "Expected Value"=w172, "Tolerance"=w173, "Samples To Average"=w175, "error in (no error)"=w181, "DAQ Channel 2"=w171, "Log"=w178, "Test Scenario"=w177, "Resistance"=w174, "Signal Name"="DAC_A Output") -> ("Constant Analog Output Voltage Test  out"=w179:refnum<class "Constant Current Output Test.lvclass">, "error out"=w180:errorcluster)  [unwired: 7 in]
        }
        frame "Verify DAC_A = 1.00A" {
          n27 = Unbundle By Name(w190) -> ("DAQ Channel 1 to Read"=w184:refnum<k21>, "DAQ Channel 2 to Read"=w185:refnum<k21>, "Expected Value"=w186:dbl, "Tolerance"=w187:dbl, "Resistor Ohms"=w188:dbl, "Samples To Average"=w189:i32)
          n28 = call "init.vi"("Constant Analog Output Voltage Test in"=refnum<class "Constant Current Output Test.lvclass"> refnum ("Constant Current Output Test.lvclass"), "DAQ Channel 1"=w184, "Expected Value"=w186, "Tolerance"=w187, "Samples To Average"=w189, "error in (no error)"=w195, "DAQ Channel 2"=w185, "Log"=w192, "Test Scenario"=w191, "Resistance"=w188, "Signal Name"="DAC_A Output") -> ("Constant Analog Output Voltage Test  out"=w193:refnum<class "Constant Current Output Test.lvclass">, "error out"=w194:errorcluster)  [unwired: 7 in]
        }
        frame "Verify DAC_B = -1.00A" {
          n29 = Unbundle By Name(w204) -> ("DAQ Channel 1 to Read"=w198:refnum<k21>, "DAQ Channel 2 to Read"=w199:refnum<k21>, "Expected Value"=w200:dbl, "Tolerance"=w201:dbl, "Resistor Ohms"=w202:dbl, "Samples To Average"=w203:i32)
          n30 = call "init.vi"("Constant Analog Output Voltage Test in"=refnum<class "Constant Current Output Test.lvclass"> refnum ("Constant Current Output Test.lvclass"), "DAQ Channel 1"=w198, "Expected Value"=w200, "Tolerance"=w201, "Samples To Average"=w203, "error in (no error)"=w209, "DAQ Channel 2"=w199, "Log"=w206, "Test Scenario"=w205, "Resistance"=w202, "Signal Name"="DAC_B Output") -> ("Constant Analog Output Voltage Test  out"=w207:refnum<class "Constant Current Output Test.lvclass">, "error out"=w208:errorcluster)  [unwired: 7 in]
        }
        frame "Verify DAC_B = -0.75A" {
          n31 = Unbundle By Name(w218) -> ("DAQ Channel 1 to Read"=w212:refnum<k21>, "DAQ Channel 2 to Read"=w213:refnum<k21>, "Expected Value"=w214:dbl, "Tolerance"=w215:dbl, "Resistor Ohms"=w216:dbl, "Samples To Average"=w217:i32)
          n32 = call "init.vi"("Constant Analog Output Voltage Test in"=refnum<class "Constant Current Output Test.lvclass"> refnum ("Constant Current Output Test.lvclass"), "DAQ Channel 1"=w212, "Expected Value"=w214, "Tolerance"=w215, "Samples To Average"=w217, "error in (no error)"=w223, "DAQ Channel 2"=w213, "Log"=w220, "Test Scenario"=w219, "Resistance"=w216, "Signal Name"="DAC_B Output") -> ("Constant Analog Output Voltage Test  out"=w221:refnum<class "Constant Current Output Test.lvclass">, "error out"=w222:errorcluster)  [unwired: 7 in]
        }
        frame "Verify DAC_B = -0.50A" {
          n33 = Unbundle By Name(w232) -> ("DAQ Channel 1 to Read"=w226:refnum<k21>, "DAQ Channel 2 to Read"=w227:refnum<k21>, "Expected Value"=w228:dbl, "Tolerance"=w229:dbl, "Resistor Ohms"=w230:dbl, "Samples To Average"=w231:i32)
          n34 = call "init.vi"("Constant Analog Output Voltage Test in"=refnum<class "Constant Current Output Test.lvclass"> refnum ("Constant Current Output Test.lvclass"), "DAQ Channel 1"=w226, "Expected Value"=w228, "Tolerance"=w229, "Samples To Average"=w231, "error in (no error)"=w237, "DAQ Channel 2"=w227, "Log"=w234, "Test Scenario"=w233, "Resistance"=w230, "Signal Name"="DAC_B Output") -> ("Constant Analog Output Voltage Test  out"=w235:refnum<class "Constant Current Output Test.lvclass">, "error out"=w236:errorcluster)  [unwired: 7 in]
        }
        frame "Verify DAC_B = -0.25A" {
          n35 = Unbundle By Name(w246) -> ("DAQ Channel 1 to Read"=w240:refnum<k21>, "DAQ Channel 2 to Read"=w241:refnum<k21>, "Expected Value"=w242:dbl, "Tolerance"=w243:dbl, "Resistor Ohms"=w244:dbl, "Samples To Average"=w245:i32)
          n36 = call "init.vi"("Constant Analog Output Voltage Test in"=refnum<class "Constant Current Output Test.lvclass"> refnum ("Constant Current Output Test.lvclass"), "DAQ Channel 1"=w240, "Expected Value"=w242, "Tolerance"=w243, "Samples To Average"=w245, "error in (no error)"=w251, "DAQ Channel 2"=w241, "Log"=w248, "Test Scenario"=w247, "Resistance"=w244, "Signal Name"="DAC_B Output") -> ("Constant Analog Output Voltage Test  out"=w249:refnum<class "Constant Current Output Test.lvclass">, "error out"=w250:errorcluster)  [unwired: 7 in]
        }
        frame "Verify DAC_B = 0.00A" {
          n37 = Unbundle By Name(w260) -> ("DAQ Channel 1 to Read"=w254:refnum<k21>, "DAQ Channel 2 to Read"=w255:refnum<k21>, "Expected Value"=w256:dbl, "Tolerance"=w257:dbl, "Resistor Ohms"=w258:dbl, "Samples To Average"=w259:i32)
          n38 = call "init.vi"("Constant Analog Output Voltage Test in"=refnum<class "Constant Current Output Test.lvclass"> refnum ("Constant Current Output Test.lvclass"), "DAQ Channel 1"=w254, "Expected Value"=w256, "Tolerance"=w257, "Samples To Average"=w259, "error in (no error)"=w265, "DAQ Channel 2"=w255, "Log"=w262, "Test Scenario"=w261, "Resistance"=w258, "Signal Name"="DAC_B Output") -> ("Constant Analog Output Voltage Test  out"=w263:refnum<class "Constant Current Output Test.lvclass">, "error out"=w264:errorcluster)  [unwired: 7 in]
        }
        frame "Verify DAC_B = 0.25A" {
          n39 = Unbundle By Name(w274) -> ("DAQ Channel 1 to Read"=w268:refnum<k21>, "DAQ Channel 2 to Read"=w269:refnum<k21>, "Expected Value"=w270:dbl, "Tolerance"=w271:dbl, "Resistor Ohms"=w272:dbl, "Samples To Average"=w273:i32)
          n40 = call "init.vi"("Constant Analog Output Voltage Test in"=refnum<class "Constant Current Output Test.lvclass"> refnum ("Constant Current Output Test.lvclass"), "DAQ Channel 1"=w268, "Expected Value"=w270, "Tolerance"=w271, "Samples To Average"=w273, "error in (no error)"=w279, "DAQ Channel 2"=w269, "Log"=w276, "Test Scenario"=w275, "Resistance"=w272, "Signal Name"="DAC_B Output") -> ("Constant Analog Output Voltage Test  out"=w277:refnum<class "Constant Current Output Test.lvclass">, "error out"=w278:errorcluster)  [unwired: 7 in]
        }
        frame "Verify DAC_B = 0.50A" {
          n41 = Unbundle By Name(w288) -> ("DAQ Channel 1 to Read"=w282:refnum<k21>, "DAQ Channel 2 to Read"=w283:refnum<k21>, "Expected Value"=w284:dbl, "Tolerance"=w285:dbl, "Resistor Ohms"=w286:dbl, "Samples To Average"=w287:i32)
          n42 = call "init.vi"("Constant Analog Output Voltage Test in"=refnum<class "Constant Current Output Test.lvclass"> refnum ("Constant Current Output Test.lvclass"), "DAQ Channel 1"=w282, "Expected Value"=w284, "Tolerance"=w285, "Samples To Average"=w287, "error in (no error)"=w293, "DAQ Channel 2"=w283, "Log"=w290, "Test Scenario"=w289, "Resistance"=w286, "Signal Name"="DAC_B Output") -> ("Constant Analog Output Voltage Test  out"=w291:refnum<class "Constant Current Output Test.lvclass">, "error out"=w292:errorcluster)  [unwired: 7 in]
        }
        frame "Verify DAC_B = 0.75A" {
          n43 = Unbundle By Name(w302) -> ("DAQ Channel 1 to Read"=w296:refnum<k21>, "DAQ Channel 2 to Read"=w297:refnum<k21>, "Expected Value"=w298:dbl, "Tolerance"=w299:dbl, "Resistor Ohms"=w300:dbl, "Samples To Average"=w301:i32)
          n44 = call "init.vi"("Constant Analog Output Voltage Test in"=refnum<class "Constant Current Output Test.lvclass"> refnum ("Constant Current Output Test.lvclass"), "DAQ Channel 1"=w296, "Expected Value"=w298, "Tolerance"=w299, "Samples To Average"=w301, "error in (no error)"=w307, "DAQ Channel 2"=w297, "Log"=w304, "Test Scenario"=w303, "Resistance"=w300, "Signal Name"="DAC_B Output") -> ("Constant Analog Output Voltage Test  out"=w305:refnum<class "Constant Current Output Test.lvclass">, "error out"=w306:errorcluster)  [unwired: 7 in]
        }
        frame "Verify DAC_B = 1.00A" {
          n45 = Unbundle By Name(w316) -> ("DAQ Channel 1 to Read"=w310:refnum<k21>, "DAQ Channel 2 to Read"=w311:refnum<k21>, "Expected Value"=w312:dbl, "Tolerance"=w313:dbl, "Resistor Ohms"=w314:dbl, "Samples To Average"=w315:i32)
          n46 = call "init.vi"("Constant Analog Output Voltage Test in"=refnum<class "Constant Current Output Test.lvclass"> refnum ("Constant Current Output Test.lvclass"), "DAQ Channel 1"=w310, "Expected Value"=w312, "Tolerance"=w313, "Samples To Average"=w315, "error in (no error)"=w321, "DAQ Channel 2"=w311, "Log"=w318, "Test Scenario"=w317, "Resistance"=w314, "Signal Name"="DAC_B Output") -> ("Constant Analog Output Voltage Test  out"=w319:refnum<class "Constant Current Output Test.lvclass">, "error out"=w320:errorcluster)  [unwired: 7 in]
        }
        frame "Set DAC_A = -1.00A" {
          n47 = Unbundle By Name(w324) -> ("Command Value"=w323:u16)
          n48 = call "init.vi"("Digital Input Test in"=refnum<class "Set ILC Test.lvclass"> refnum ("Set DAC Test.lvclass"), "Command"=w323, "ConfigureILCStrategy"=refnum<class "ConfigureILCDCADAC1Strategy.lvclass"> refnum ("ConfigureILCDCADAC1Strategy.lvclass"), "error in (no error)"=w328, "Test Scenario"=w329, "Log"=w326, "Signal Name"="Set DAC_A") -> ("Digital Input Test out"=w331:refnum<class "Set ILC Test.lvclass">, "error out"=w327:errorcluster)  [unwired: 11 in]
        }
        frame "Set DAC_A = -0.75A" {
          n49 = Unbundle By Name(w334) -> ("Command Value"=w333:u16)
          n50 = call "init.vi"("Digital Input Test in"=refnum<class "Set ILC Test.lvclass"> refnum ("Set DAC Test.lvclass"), "Command"=w333, "ConfigureILCStrategy"=refnum<class "ConfigureILCDCADAC1Strategy.lvclass"> refnum ("ConfigureILCDCADAC1Strategy.lvclass"), "error in (no error)"=w338, "Test Scenario"=w339, "Log"=w336, "Signal Name"="Set DAC_A") -> ("Digital Input Test out"=w341:refnum<class "Set ILC Test.lvclass">, "error out"=w337:errorcluster)  [unwired: 11 in]
        }
        frame "Set DAC_A = -0.50A" {
          n51 = Unbundle By Name(w344) -> ("Command Value"=w343:u16)
          n52 = call "init.vi"("Digital Input Test in"=refnum<class "Set ILC Test.lvclass"> refnum ("Set DAC Test.lvclass"), "Command"=w343, "ConfigureILCStrategy"=refnum<class "ConfigureILCDCADAC1Strategy.lvclass"> refnum ("ConfigureILCDCADAC1Strategy.lvclass"), "error in (no error)"=w348, "Test Scenario"=w349, "Log"=w346, "Signal Name"="Set DAC_A") -> ("Digital Input Test out"=w351:refnum<class "Set ILC Test.lvclass">, "error out"=w347:errorcluster)  [unwired: 11 in]
        }
        frame "Set DAC_A = -0.25A" {
          n53 = Unbundle By Name(w354) -> ("Command Value"=w353:u16)
          n54 = call "init.vi"("Digital Input Test in"=refnum<class "Set ILC Test.lvclass"> refnum ("Set DAC Test.lvclass"), "Command"=w353, "ConfigureILCStrategy"=refnum<class "ConfigureILCDCADAC1Strategy.lvclass"> refnum ("ConfigureILCDCADAC1Strategy.lvclass"), "error in (no error)"=w358, "Test Scenario"=w359, "Log"=w356, "Signal Name"="Set DAC_A") -> ("Digital Input Test out"=w361:refnum<class "Set ILC Test.lvclass">, "error out"=w357:errorcluster)  [unwired: 11 in]
        }
        frame "Set DAC_A = 0.00A" {
          n55 = Unbundle By Name(w364) -> ("Command Value"=w363:u16)
          n56 = call "init.vi"("Digital Input Test in"=refnum<class "Set ILC Test.lvclass"> refnum ("Set DAC Test.lvclass"), "Command"=w363, "ConfigureILCStrategy"=refnum<class "ConfigureILCDCADAC1Strategy.lvclass"> refnum ("ConfigureILCDCADAC1Strategy.lvclass"), "error in (no error)"=w368, "Test Scenario"=w369, "Log"=w366, "Signal Name"="Set DAC_A") -> ("Digital Input Test out"=w371:refnum<class "Set ILC Test.lvclass">, "error out"=w367:errorcluster)  [unwired: 11 in]
        }
        frame "Set DAC_A = 0.25A" {
          n57 = Unbundle By Name(w374) -> ("Command Value"=w373:u16)
          n58 = call "init.vi"("Digital Input Test in"=refnum<class "Set ILC Test.lvclass"> refnum ("Set DAC Test.lvclass"), "Command"=w373, "ConfigureILCStrategy"=refnum<class "ConfigureILCDCADAC1Strategy.lvclass"> refnum ("ConfigureILCDCADAC1Strategy.lvclass"), "error in (no error)"=w378, "Test Scenario"=w379, "Log"=w376, "Signal Name"="Set DAC_A") -> ("Digital Input Test out"=w381:refnum<class "Set ILC Test.lvclass">, "error out"=w377:errorcluster)  [unwired: 11 in]
        }
        frame "Set DAC_A = 0.50A" {
          n59 = Unbundle By Name(w384) -> ("Command Value"=w383:u16)
          n60 = call "init.vi"("Digital Input Test in"=refnum<class "Set ILC Test.lvclass"> refnum ("Set DAC Test.lvclass"), "Command"=w383, "ConfigureILCStrategy"=refnum<class "ConfigureILCDCADAC1Strategy.lvclass"> refnum ("ConfigureILCDCADAC1Strategy.lvclass"), "error in (no error)"=w388, "Test Scenario"=w389, "Log"=w386, "Signal Name"="Set DAC_A") -> ("Digital Input Test out"=w391:refnum<class "Set ILC Test.lvclass">, "error out"=w387:errorcluster)  [unwired: 11 in]
        }
        frame "Set DAC_A = 0.75A" {
          n61 = Unbundle By Name(w394) -> ("Command Value"=w393:u16)
          n62 = call "init.vi"("Digital Input Test in"=refnum<class "Set ILC Test.lvclass"> refnum ("Set DAC Test.lvclass"), "Command"=w393, "ConfigureILCStrategy"=refnum<class "ConfigureILCDCADAC1Strategy.lvclass"> refnum ("ConfigureILCDCADAC1Strategy.lvclass"), "error in (no error)"=w398, "Test Scenario"=w399, "Log"=w396, "Signal Name"="Set DAC_A") -> ("Digital Input Test out"=w401:refnum<class "Set ILC Test.lvclass">, "error out"=w397:errorcluster)  [unwired: 11 in]
        }
        frame "Set DAC_A = 1.00A" {
          n63 = Unbundle By Name(w404) -> ("Command Value"=w403:u16)
          n64 = call "init.vi"("Digital Input Test in"=refnum<class "Set ILC Test.lvclass"> refnum ("Set DAC Test.lvclass"), "Command"=w403, "ConfigureILCStrategy"=refnum<class "ConfigureILCDCADAC1Strategy.lvclass"> refnum ("ConfigureILCDCADAC1Strategy.lvclass"), "error in (no error)"=w408, "Test Scenario"=w409, "Log"=w406, "Signal Name"="Set DAC_A") -> ("Digital Input Test out"=w411:refnum<class "Set ILC Test.lvclass">, "error out"=w407:errorcluster)  [unwired: 11 in]
        }
        frame "Set DAC_B = -1.00A" {
          n65 = Unbundle By Name(w415) -> ("Command Value"=w414:u16)
          n66 = call "init.vi"("Digital Input Test in"=refnum<class "Set ILC Test.lvclass"> refnum ("Set DAC Test.lvclass"), "Command"=w414, "ConfigureILCStrategy"=refnum<class "ConfigureILCDCADAC2Strategy.lvclass"> refnum ("ConfigureILCDCADAC2Strategy.lvclass"), "error in (no error)"=w418, "Test Scenario"=w419, "Log"=w416, "Signal Name"="Set DAC_B") -> ("Digital Input Test out"=w421:refnum<class "Set ILC Test.lvclass">, "error out"=w417:errorcluster)  [unwired: 11 in]
        }
        frame "Set DAC_B = -0.75A" {
          n67 = Unbundle By Name(w425) -> ("Command Value"=w424:u16)
          n68 = call "init.vi"("Digital Input Test in"=refnum<class "Set ILC Test.lvclass"> refnum ("Set DAC Test.lvclass"), "Command"=w424, "ConfigureILCStrategy"=refnum<class "ConfigureILCDCADAC2Strategy.lvclass"> refnum ("ConfigureILCDCADAC2Strategy.lvclass"), "error in (no error)"=w428, "Test Scenario"=w429, "Log"=w426, "Signal Name"="Set DAC_B") -> ("Digital Input Test out"=w431:refnum<class "Set ILC Test.lvclass">, "error out"=w427:errorcluster)  [unwired: 11 in]
        }
        frame "Set DAC_B = -0.50A" {
          n69 = Unbundle By Name(w435) -> ("Command Value"=w434:u16)
          n70 = call "init.vi"("Digital Input Test in"=refnum<class "Set ILC Test.lvclass"> refnum ("Set DAC Test.lvclass"), "Command"=w434, "ConfigureILCStrategy"=refnum<class "ConfigureILCDCADAC2Strategy.lvclass"> refnum ("ConfigureILCDCADAC2Strategy.lvclass"), "error in (no error)"=w438, "Test Scenario"=w439, "Log"=w436, "Signal Name"="Set DAC_B") -> ("Digital Input Test out"=w441:refnum<class "Set ILC Test.lvclass">, "error out"=w437:errorcluster)  [unwired: 11 in]
        }
        frame "Set DAC_B = -0.25A" {
          n71 = Unbundle By Name(w445) -> ("Command Value"=w444:u16)
          n72 = call "init.vi"("Digital Input Test in"=refnum<class "Set ILC Test.lvclass"> refnum ("Set DAC Test.lvclass"), "Command"=w444, "ConfigureILCStrategy"=refnum<class "ConfigureILCDCADAC2Strategy.lvclass"> refnum ("ConfigureILCDCADAC2Strategy.lvclass"), "error in (no error)"=w448, "Test Scenario"=w449, "Log"=w446, "Signal Name"="Set DAC_B") -> ("Digital Input Test out"=w451:refnum<class "Set ILC Test.lvclass">, "error out"=w447:errorcluster)  [unwired: 11 in]
        }
        frame "Set DAC_B = 0.00A" {
          n73 = Unbundle By Name(w455) -> ("Command Value"=w454:u16)
          n74 = call "init.vi"("Digital Input Test in"=refnum<class "Set ILC Test.lvclass"> refnum ("Set DAC Test.lvclass"), "Command"=w454, "ConfigureILCStrategy"=refnum<class "ConfigureILCDCADAC2Strategy.lvclass"> refnum ("ConfigureILCDCADAC2Strategy.lvclass"), "error in (no error)"=w458, "Test Scenario"=w459, "Log"=w456, "Signal Name"="Set DAC_B") -> ("Digital Input Test out"=w461:refnum<class "Set ILC Test.lvclass">, "error out"=w457:errorcluster)  [unwired: 11 in]
        }
        frame "Set DAC_B = 0.25A" {
          n75 = Unbundle By Name(w465) -> ("Command Value"=w464:u16)
          n76 = call "init.vi"("Digital Input Test in"=refnum<class "Set ILC Test.lvclass"> refnum ("Set DAC Test.lvclass"), "Command"=w464, "ConfigureILCStrategy"=refnum<class "ConfigureILCDCADAC2Strategy.lvclass"> refnum ("ConfigureILCDCADAC2Strategy.lvclass"), "error in (no error)"=w468, "Test Scenario"=w469, "Log"=w466, "Signal Name"="Set DAC_B") -> ("Digital Input Test out"=w471:refnum<class "Set ILC Test.lvclass">, "error out"=w467:errorcluster)  [unwired: 11 in]
        }
        frame "Set DAC_B = 0.50A" {
          n77 = Unbundle By Name(w475) -> ("Command Value"=w474:u16)
          n78 = call "init.vi"("Digital Input Test in"=refnum<class "Set ILC Test.lvclass"> refnum ("Set DAC Test.lvclass"), "Command"=w474, "ConfigureILCStrategy"=refnum<class "ConfigureILCDCADAC2Strategy.lvclass"> refnum ("ConfigureILCDCADAC2Strategy.lvclass"), "error in (no error)"=w478, "Test Scenario"=w479, "Log"=w476, "Signal Name"="Set DAC_B") -> ("Digital Input Test out"=w481:refnum<class "Set ILC Test.lvclass">, "error out"=w477:errorcluster)  [unwired: 11 in]
        }
        frame "Set DAC_B = 0.75A" {
          n79 = Unbundle By Name(w485) -> ("Command Value"=w484:u16)
          n80 = call "init.vi"("Digital Input Test in"=refnum<class "Set ILC Test.lvclass"> refnum ("Set DAC Test.lvclass"), "Command"=w484, "ConfigureILCStrategy"=refnum<class "ConfigureILCDCADAC2Strategy.lvclass"> refnum ("ConfigureILCDCADAC2Strategy.lvclass"), "error in (no error)"=w488, "Test Scenario"=w489, "Log"=w486, "Signal Name"="Set DAC_B") -> ("Digital Input Test out"=w491:refnum<class "Set ILC Test.lvclass">, "error out"=w487:errorcluster)  [unwired: 11 in]
        }
        frame "Set DAC_B = 1.00A" {
          n81 = Unbundle By Name(w495) -> ("Command Value"=w494:u16)
          n82 = call "init.vi"("Digital Input Test in"=refnum<class "Set ILC Test.lvclass"> refnum ("Set DAC Test.lvclass"), "Command"=w494, "ConfigureILCStrategy"=refnum<class "ConfigureILCDCADAC2Strategy.lvclass"> refnum ("ConfigureILCDCADAC2Strategy.lvclass"), "error in (no error)"=w498, "Test Scenario"=w499, "Log"=w496, "Signal Name"="Set DAC_B") -> ("Digital Input Test out"=w501:refnum<class "Set ILC Test.lvclass">, "error out"=w497:errorcluster)  [unwired: 11 in]
        }
        frame "Set MTR_PWR = On" {
          n83 = Unbundle By Name(w505) -> ("Motor Enable"=w504:u16)
          n84 = call "init.vi"("Digital Input Test in"=refnum<class "Set ILC Test.lvclass"> refnum ("Set DAC Test.lvclass"), "Command"=w504, "ConfigureILCStrategy"=refnum<class "ConfigureILCSSRStrategy.lvclass"> refnum ("ConfigureILCSSRStrategy.lvclass"), "error in (no error)"=w508, "Test Scenario"=w509, "Log"=w506, "Signal Name"="Set MTR_PWR") -> ("Digital Input Test out"=w511:refnum<class "Set ILC Test.lvclass">, "error out"=w507:errorcluster)  [unwired: 11 in]
        }
        frame "Set MTR_PWR = Off" {
          n85 = Unbundle By Name(w515) -> ("Motor Disable"=w514:u16)
          n86 = call "init.vi"("Digital Input Test in"=refnum<class "Set ILC Test.lvclass"> refnum ("Set DAC Test.lvclass"), "Command"=w514, "ConfigureILCStrategy"=refnum<class "ConfigureILCSSRStrategy.lvclass"> refnum ("ConfigureILCSSRStrategy.lvclass"), "error in (no error)"=w518, "Test Scenario"=w519, "Log"=w516, "Signal Name"="Set MTR_PWR") -> ("Digital Input Test out"=w521:refnum<class "Set ILC Test.lvclass">, "error out"=w517:errorcluster)  [unwired: 11 in]
        }
        frame "Set OUTPUT = On" {
          n87 = Unbundle By Name(w525) -> ("Current Output Enable"=w524:u16)
          n88 = call "init.vi"("Digital Input Test in"=refnum<class "Set ILC Test.lvclass"> refnum ("Set DAC Test.lvclass"), "Command"=w524, "ConfigureILCStrategy"=refnum<class "ConfigureILCDCAOutputStrategy.lvclass"> refnum ("ConfigureILCDCAOutputStrategy.lvclass"), "error in (no error)"=w528, "Test Scenario"=w529, "Log"=w526, "Signal Name"="Set OUTPUT") -> ("Digital Input Test out"=w531:refnum<class "Set ILC Test.lvclass">, "error out"=w527:errorcluster)  [unwired: 11 in]
        }
        frame "Set OUTPUT = Off" {
          n89 = Unbundle By Name(w535) -> ("Current Output Disable"=w534:u16)
          n90 = call "init.vi"("Digital Input Test in"=refnum<class "Set ILC Test.lvclass"> refnum ("Set DAC Test.lvclass"), "Command"=w534, "ConfigureILCStrategy"=refnum<class "ConfigureILCDCAOutputStrategy.lvclass"> refnum ("ConfigureILCDCAOutputStrategy.lvclass"), "error in (no error)"=w538, "Test Scenario"=w539, "Log"=w536, "Signal Name"="Set OUTPUT") -> ("Digital Input Test out"=w541:refnum<class "Set ILC Test.lvclass">, "error out"=w537:errorcluster)  [unwired: 11 in]
        }
        frame "Verify OUTPUT = On" {
          n91 = Unbundle By Name(w553) -> ("Current Output Enable"=w543:u16)
          n92 = call "init.vi"("Digital Input Test in"=refnum<class "Verify ILC Test.lvclass"> refnum ("Verify ILC Test.lvclass"), "ReadILCStrategy"=refnum<class "ReadILCDCAOutputStrategy.lvclass"> refnum ("ReadILCDCAOutputStrategy.lvclass"), "ConfigureILCStrategy"=refnum<class "ConfigureILCDCAPressureStrategy.lvclass"> refnum ("ConfigureILCDCAPressureStrategy.lvclass"), "Expected"=w543, "Tolerance"=0.0, "error in (no error)"=w549, "Test Scenario"=w548, "Log"=w547, "Signal Name"="OUTPUT") -> ("Digital Input Test out"=w551:refnum<class "Verify ILC Test.lvclass">, "error out"=w550:errorcluster)  [unwired: 9 in]
        }
        frame "Verify OUTPUT = Off" {
          n93 = Unbundle By Name(w565) -> ("Current Output Disable"=w555:u16)
          n94 = call "init.vi"("Digital Input Test in"=refnum<class "Verify ILC Test.lvclass"> refnum ("Verify ILC Test.lvclass"), "ReadILCStrategy"=refnum<class "ReadILCDCAOutputStrategy.lvclass"> refnum ("ReadILCDCAOutputStrategy.lvclass"), "ConfigureILCStrategy"=refnum<class "ConfigureILCDCAPressureStrategy.lvclass"> refnum ("ConfigureILCDCAPressureStrategy.lvclass"), "Expected"=w555, "Tolerance"=0.0, "error in (no error)"=w561, "Test Scenario"=w560, "Log"=w559, "Signal Name"="OUTPUT") -> ("Digital Input Test out"=w563:refnum<class "Verify ILC Test.lvclass">, "error out"=w562:errorcluster)  [unwired: 9 in]
        }
        frame "Verify POWER = Ok" {
          n95 = Unbundle By Name(w577) -> ("Power Enable"=w568:u16)
          n96 = call "init.vi"("Digital Input Test in"=refnum<class "Verify ILC Test.lvclass"> refnum ("Verify ILC Test.lvclass"), "ReadILCStrategy"=refnum<class "ReadILCDCAPowerFailStrategy.lvclass"> refnum ("ReadILCDCAPowerFailStrategy.lvclass"), "ConfigureILCStrategy"=refnum<class "ConfigureILCDCAPressureStrategy.lvclass"> refnum ("ConfigureILCDCAPressureStrategy.lvclass"), "Expected"=w568, "Tolerance"=0.0, "error in (no error)"=w573, "Test Scenario"=w572, "Log"=w571, "Signal Name"="POWER") -> ("Digital Input Test out"=w575:refnum<class "Verify ILC Test.lvclass">, "error out"=w574:errorcluster)  [unwired: 9 in]
        }
        frame "Verify POWER = Fail" {
          n97 = Unbundle By Name(w589) -> ("Power Disable"=w580:u16)
          n98 = call "init.vi"("Digital Input Test in"=refnum<class "Verify ILC Test.lvclass"> refnum ("Verify ILC Test.lvclass"), "ReadILCStrategy"=refnum<class "ReadILCDCAPowerFailStrategy.lvclass"> refnum ("ReadILCDCAPowerFailStrategy.lvclass"), "ConfigureILCStrategy"=refnum<class "ConfigureILCDCAPressureStrategy.lvclass"> refnum ("ConfigureILCDCAPressureStrategy.lvclass"), "Expected"=w580, "Tolerance"=0.0, "error in (no error)"=w585, "Test Scenario"=w584, "Log"=w583, "Signal Name"="POWER") -> ("Digital Input Test out"=w587:refnum<class "Verify ILC Test.lvclass">, "error out"=w586:errorcluster)  [unwired: 9 in]
        }
        frame "Verify AMP1 = Ok" {
          n99 = Unbundle By Name(w601) -> ("Amplifier Enable"=w592:u16)
          n100 = call "init.vi"("Digital Input Test in"=refnum<class "Verify ILC Test.lvclass"> refnum ("Verify ILC Test.lvclass"), "ReadILCStrategy"=refnum<class "ReadILCDCAAmp1FailStrategy.lvclass"> refnum ("ReadILCDCAAmp1FailStrategy.lvclass"), "ConfigureILCStrategy"=refnum<class "ConfigureILCDCAPressureStrategy.lvclass"> refnum ("ConfigureILCDCAPressureStrategy.lvclass"), "Expected"=w592, "Tolerance"=0.0, "error in (no error)"=w597, "Test Scenario"=w596, "Log"=w595, "Signal Name"="AMP1") -> ("Digital Input Test out"=w599:refnum<class "Verify ILC Test.lvclass">, "error out"=w598:errorcluster)  [unwired: 9 in]
        }
        frame "Verify AMP1 = Fail" {
          n101 = Unbundle By Name(w613) -> ("Amplifier Disable"=w604:u16)
          n102 = call "init.vi"("Digital Input Test in"=refnum<class "Verify ILC Test.lvclass"> refnum ("Verify ILC Test.lvclass"), "ReadILCStrategy"=refnum<class "ReadILCDCAAmp1FailStrategy.lvclass"> refnum ("ReadILCDCAAmp1FailStrategy.lvclass"), "ConfigureILCStrategy"=refnum<class "ConfigureILCDCAPressureStrategy.lvclass"> refnum ("ConfigureILCDCAPressureStrategy.lvclass"), "Expected"=w604, "Tolerance"=0.0, "error in (no error)"=w609, "Test Scenario"=w608, "Log"=w607, "Signal Name"="AMP1") -> ("Digital Input Test out"=w611:refnum<class "Verify ILC Test.lvclass">, "error out"=w610:errorcluster)  [unwired: 9 in]
        }
        frame "Verify AMP2 = Ok" {
          n103 = Unbundle By Name(w625) -> ("Amplifier Enable"=w616:u16)
          n104 = call "init.vi"("Digital Input Test in"=refnum<class "Verify ILC Test.lvclass"> refnum ("Verify ILC Test.lvclass"), "ReadILCStrategy"=refnum<class "ReadILCDCAAmp2FailStrategy.lvclass"> refnum ("ReadILCDCAAmp2FailStrategy.lvclass"), "ConfigureILCStrategy"=refnum<class "ConfigureILCDCAPressureStrategy.lvclass"> refnum ("ConfigureILCDCAPressureStrategy.lvclass"), "Expected"=w616, "Tolerance"=0.0, "error in (no error)"=w621, "Test Scenario"=w620, "Log"=w619, "Signal Name"="AMP2") -> ("Digital Input Test out"=w623:refnum<class "Verify ILC Test.lvclass">, "error out"=w622:errorcluster)  [unwired: 9 in]
        }
        frame "Verify AMP2 = Fail" {
          n105 = Unbundle By Name(w637) -> ("Amplifier Disable"=w628:u16)
          n106 = call "init.vi"("Digital Input Test in"=refnum<class "Verify ILC Test.lvclass"> refnum ("Verify ILC Test.lvclass"), "ReadILCStrategy"=refnum<class "ReadILCDCAAmp2FailStrategy.lvclass"> refnum ("ReadILCDCAAmp2FailStrategy.lvclass"), "ConfigureILCStrategy"=refnum<class "ConfigureILCDCAPressureStrategy.lvclass"> refnum ("ConfigureILCDCAPressureStrategy.lvclass"), "Expected"=w628, "Tolerance"=0.0, "error in (no error)"=w633, "Test Scenario"=w632, "Log"=w631, "Signal Name"="AMP2") -> ("Digital Input Test out"=w635:refnum<class "Verify ILC Test.lvclass">, "error out"=w634:errorcluster)  [unwired: 9 in]
        }
        frame "P1 0%" {
          n107 = Unbundle By Name(w642) -> ("Samples To Average"=w641:i32, "Settling (ms)"=w640:u16, "Delay (ms)"=w639:u16, "0% Test"=w638:T2)
          n108 = call "init.vi"("Digital Input Test in"=refnum<class "Test Pressure.lvclass"> refnum ("Test Pressure.lvclass"), "ReadILCStrategy"=refnum<class "ReadILCDCAPressure1Strategy.lvclass"> refnum ("ReadILCDCAPressure1Strategy.lvclass"), "ConfigureILCStrategy"=refnum<class "ConfigureILCDAC1Strategy.lvclass"> refnum ("ConfigureILCDAC1Strategy.lvclass"), "Pressure Test"=w638, "Sample Delay"=w639, "error in (no error)"=w649, "Test Scenario"=w647, "Log"=w646, "Signal Name"="P1", "Wait"=w640, "Samples To Read"=w641) -> ("Digital Input Test out"=w650:refnum<class "Test Pressure.lvclass">, "error out"=w648:errorcluster)  [unwired: 7 in]
        }
        frame "P1 25%" {
          n109 = Unbundle By Name(w656) -> ("Samples To Average"=w655:i32, "Settling (ms)"=w654:u16, "Delay (ms)"=w653:u16, "25% Test"=w652:T2)
          n110 = call "init.vi"("Digital Input Test in"=refnum<class "Test Pressure.lvclass"> refnum ("Test Pressure.lvclass"), "ReadILCStrategy"=refnum<class "ReadILCDCAPressure1Strategy.lvclass"> refnum ("ReadILCDCAPressure1Strategy.lvclass"), "ConfigureILCStrategy"=refnum<class "ConfigureILCDAC1Strategy.lvclass"> refnum ("ConfigureILCDAC1Strategy.lvclass"), "Pressure Test"=w652, "Sample Delay"=w653, "error in (no error)"=w663, "Test Scenario"=w661, "Log"=w660, "Signal Name"="P1", "Wait"=w654, "Samples To Read"=w655) -> ("Digital Input Test out"=w664:refnum<class "Test Pressure.lvclass">, "error out"=w662:errorcluster)  [unwired: 7 in]
        }
        frame "P1 50%" {
          n111 = Unbundle By Name(w670) -> ("Samples To Average"=w669:i32, "Settling (ms)"=w668:u16, "Delay (ms)"=w667:u16, "50% Test"=w666:T2)
          n112 = call "init.vi"("Digital Input Test in"=refnum<class "Test Pressure.lvclass"> refnum ("Test Pressure.lvclass"), "ReadILCStrategy"=refnum<class "ReadILCDCAPressure1Strategy.lvclass"> refnum ("ReadILCDCAPressure1Strategy.lvclass"), "ConfigureILCStrategy"=refnum<class "ConfigureILCDAC1Strategy.lvclass"> refnum ("ConfigureILCDAC1Strategy.lvclass"), "Pressure Test"=w666, "Sample Delay"=w667, "error in (no error)"=w677, "Test Scenario"=w675, "Log"=w674, "Signal Name"="P1", "Wait"=w668, "Samples To Read"=w669) -> ("Digital Input Test out"=w678:refnum<class "Test Pressure.lvclass">, "error out"=w676:errorcluster)  [unwired: 7 in]
        }
        frame "P1 75%" {
          n113 = Unbundle By Name(w684) -> ("Samples To Average"=w683:i32, "Settling (ms)"=w682:u16, "Delay (ms)"=w681:u16, "75% Test"=w680:T2)
          n114 = call "init.vi"("Digital Input Test in"=refnum<class "Test Pressure.lvclass"> refnum ("Test Pressure.lvclass"), "ReadILCStrategy"=refnum<class "ReadILCDCAPressure1Strategy.lvclass"> refnum ("ReadILCDCAPressure1Strategy.lvclass"), "ConfigureILCStrategy"=refnum<class "ConfigureILCDAC1Strategy.lvclass"> refnum ("ConfigureILCDAC1Strategy.lvclass"), "Pressure Test"=w680, "Sample Delay"=w681, "error in (no error)"=w691, "Test Scenario"=w689, "Log"=w688, "Signal Name"="P1", "Wait"=w682, "Samples To Read"=w683) -> ("Digital Input Test out"=w692:refnum<class "Test Pressure.lvclass">, "error out"=w690:errorcluster)  [unwired: 7 in]
        }
        frame "P1 100%" {
          n115 = Unbundle By Name(w698) -> ("Samples To Average"=w697:i32, "Settling (ms)"=w696:u16, "Delay (ms)"=w695:u16, "100% Test"=w694:T2)
          n116 = call "init.vi"("Digital Input Test in"=refnum<class "Test Pressure.lvclass"> refnum ("Test Pressure.lvclass"), "ReadILCStrategy"=refnum<class "ReadILCDCAPressure1Strategy.lvclass"> refnum ("ReadILCDCAPressure1Strategy.lvclass"), "ConfigureILCStrategy"=refnum<class "ConfigureILCDAC1Strategy.lvclass"> refnum ("ConfigureILCDAC1Strategy.lvclass"), "Pressure Test"=w694, "Sample Delay"=w695, "error in (no error)"=w705, "Test Scenario"=w703, "Log"=w702, "Signal Name"="P1", "Wait"=w696, "Samples To Read"=w697) -> ("Digital Input Test out"=w706:refnum<class "Test Pressure.lvclass">, "error out"=w704:errorcluster)  [unwired: 7 in]
        }
        frame "P2 0%" {
          n117 = Unbundle By Name(w714) -> ("Samples To Average"=w713:i32, "Settling (ms)"=w712:u16, "Delay (ms)"=w711:u16, "0% Test"=w710:T2)
          n118 = call "init.vi"("Digital Input Test in"=refnum<class "Test Pressure.lvclass"> refnum ("Test Pressure.lvclass"), "ReadILCStrategy"=refnum<class "ReadILCDCAPressure2Strategy.lvclass"> refnum ("ReadILCDCAPressure2Strategy.lvclass"), "ConfigureILCStrategy"=refnum<class "ConfigureILCDAC2Strategy.lvclass"> refnum ("ConfigureILCDAC2Strategy.lvclass"), "Pressure Test"=w710, "Sample Delay"=w711, "error in (no error)"=w719, "Test Scenario"=w717, "Log"=w716, "Signal Name"="P2", "Wait"=w712, "Samples To Read"=w713) -> ("Digital Input Test out"=w720:refnum<class "Test Pressure.lvclass">, "error out"=w718:errorcluster)  [unwired: 7 in]
        }
        frame "P2 25%" {
          n119 = Unbundle By Name(w728) -> ("Samples To Average"=w727:i32, "Settling (ms)"=w726:u16, "Delay (ms)"=w725:u16, "25% Test"=w724:T2)
          n120 = call "init.vi"("Digital Input Test in"=refnum<class "Test Pressure.lvclass"> refnum ("Test Pressure.lvclass"), "ReadILCStrategy"=refnum<class "ReadILCDCAPressure2Strategy.lvclass"> refnum ("ReadILCDCAPressure2Strategy.lvclass"), "ConfigureILCStrategy"=refnum<class "ConfigureILCDAC2Strategy.lvclass"> refnum ("ConfigureILCDAC2Strategy.lvclass"), "Pressure Test"=w724, "Sample Delay"=w725, "error in (no error)"=w733, "Test Scenario"=w731, "Log"=w730, "Signal Name"="P2", "Wait"=w726, "Samples To Read"=w727) -> ("Digital Input Test out"=w734:refnum<class "Test Pressure.lvclass">, "error out"=w732:errorcluster)  [unwired: 7 in]
        }
        frame "P2 50%" {
          n121 = Unbundle By Name(w742) -> ("Samples To Average"=w741:i32, "Settling (ms)"=w740:u16, "Delay (ms)"=w739:u16, "50% Test"=w738:T2)
          n122 = call "init.vi"("Digital Input Test in"=refnum<class "Test Pressure.lvclass"> refnum ("Test Pressure.lvclass"), "ReadILCStrategy"=refnum<class "ReadILCDCAPressure2Strategy.lvclass"> refnum ("ReadILCDCAPressure2Strategy.lvclass"), "ConfigureILCStrategy"=refnum<class "ConfigureILCDAC2Strategy.lvclass"> refnum ("ConfigureILCDAC2Strategy.lvclass"), "Pressure Test"=w738, "Sample Delay"=w739, "error in (no error)"=w747, "Test Scenario"=w745, "Log"=w744, "Signal Name"="P2", "Wait"=w740, "Samples To Read"=w741) -> ("Digital Input Test out"=w748:refnum<class "Test Pressure.lvclass">, "error out"=w746:errorcluster)  [unwired: 7 in]
        }
        frame "P2 75%" {
          n123 = Unbundle By Name(w756) -> ("Samples To Average"=w755:i32, "Settling (ms)"=w754:u16, "Delay (ms)"=w753:u16, "75% Test"=w752:T2)
          n124 = call "init.vi"("Digital Input Test in"=refnum<class "Test Pressure.lvclass"> refnum ("Test Pressure.lvclass"), "ReadILCStrategy"=refnum<class "ReadILCDCAPressure2Strategy.lvclass"> refnum ("ReadILCDCAPressure2Strategy.lvclass"), "ConfigureILCStrategy"=refnum<class "ConfigureILCDAC2Strategy.lvclass"> refnum ("ConfigureILCDAC2Strategy.lvclass"), "Pressure Test"=w752, "Sample Delay"=w753, "error in (no error)"=w761, "Test Scenario"=w759, "Log"=w758, "Signal Name"="P2", "Wait"=w754, "Samples To Read"=w755) -> ("Digital Input Test out"=w762:refnum<class "Test Pressure.lvclass">, "error out"=w760:errorcluster)  [unwired: 7 in]
        }
        frame "P2 100%" {
          n125 = Unbundle By Name(w770) -> ("Samples To Average"=w769:i32, "Settling (ms)"=w768:u16, "Delay (ms)"=w767:u16, "100% Test"=w766:T2)
          n126 = call "init.vi"("Digital Input Test in"=refnum<class "Test Pressure.lvclass"> refnum ("Test Pressure.lvclass"), "ReadILCStrategy"=refnum<class "ReadILCDCAPressure2Strategy.lvclass"> refnum ("ReadILCDCAPressure2Strategy.lvclass"), "ConfigureILCStrategy"=refnum<class "ConfigureILCDAC2Strategy.lvclass"> refnum ("ConfigureILCDAC2Strategy.lvclass"), "Pressure Test"=w766, "Sample Delay"=w767, "error in (no error)"=w775, "Test Scenario"=w773, "Log"=w772, "Signal Name"="P2", "Wait"=w768, "Samples To Read"=w769) -> ("Digital Input Test out"=w776:refnum<class "Test Pressure.lvclass">, "error out"=w774:errorcluster)  [unwired: 7 in]
        }
        frame "P3 0%" {
          n127 = Unbundle By Name(w784) -> ("Samples To Average"=w783:i32, "Settling (ms)"=w782:u16, "Delay (ms)"=w781:u16, "0% Test"=w780:T2)
          n128 = call "init.vi"("Digital Input Test in"=refnum<class "Test Pressure.lvclass"> refnum ("Test Pressure.lvclass"), "ReadILCStrategy"=refnum<class "ReadILCDCAPressure3Strategy.lvclass"> refnum ("ReadILCDCAPressure3Strategy.lvclass"), "ConfigureILCStrategy"=refnum<class "ConfigureILCDAC3Strategy.lvclass"> refnum ("ConfigureILCDAC3Strategy.lvclass"), "Pressure Test"=w780, "Sample Delay"=w781, "error in (no error)"=w789, "Test Scenario"=w787, "Log"=w786, "Signal Name"="P3", "Wait"=w782, "Samples To Read"=w783) -> ("Digital Input Test out"=w790:refnum<class "Test Pressure.lvclass">, "error out"=w788:errorcluster)  [unwired: 7 in]
        }
        frame "P3 25%" {
          n129 = Unbundle By Name(w798) -> ("Samples To Average"=w797:i32, "Settling (ms)"=w796:u16, "Delay (ms)"=w795:u16, "25% Test"=w794:T2)
          n130 = call "init.vi"("Digital Input Test in"=refnum<class "Test Pressure.lvclass"> refnum ("Test Pressure.lvclass"), "ReadILCStrategy"=refnum<class "ReadILCDCAPressure3Strategy.lvclass"> refnum ("ReadILCDCAPressure3Strategy.lvclass"), "ConfigureILCStrategy"=refnum<class "ConfigureILCDAC3Strategy.lvclass"> refnum ("ConfigureILCDAC3Strategy.lvclass"), "Pressure Test"=w794, "Sample Delay"=w795, "error in (no error)"=w803, "Test Scenario"=w801, "Log"=w800, "Signal Name"="P3", "Wait"=w796, "Samples To Read"=w797) -> ("Digital Input Test out"=w804:refnum<class "Test Pressure.lvclass">, "error out"=w802:errorcluster)  [unwired: 7 in]
        }
        frame "P3 50%" {
          n131 = Unbundle By Name(w812) -> ("Samples To Average"=w811:i32, "Settling (ms)"=w810:u16, "Delay (ms)"=w809:u16, "50% Test"=w808:T2)
          n132 = call "init.vi"("Digital Input Test in"=refnum<class "Test Pressure.lvclass"> refnum ("Test Pressure.lvclass"), "ReadILCStrategy"=refnum<class "ReadILCDCAPressure3Strategy.lvclass"> refnum ("ReadILCDCAPressure3Strategy.lvclass"), "ConfigureILCStrategy"=refnum<class "ConfigureILCDAC3Strategy.lvclass"> refnum ("ConfigureILCDAC3Strategy.lvclass"), "Pressure Test"=w808, "Sample Delay"=w809, "error in (no error)"=w817, "Test Scenario"=w815, "Log"=w814, "Signal Name"="P3", "Wait"=w810, "Samples To Read"=w811) -> ("Digital Input Test out"=w818:refnum<class "Test Pressure.lvclass">, "error out"=w816:errorcluster)  [unwired: 7 in]
        }
        frame "P3 75%" {
          n133 = Unbundle By Name(w826) -> ("Samples To Average"=w825:i32, "Settling (ms)"=w824:u16, "Delay (ms)"=w823:u16, "75% Test"=w822:T2)
          n134 = call "init.vi"("Digital Input Test in"=refnum<class "Test Pressure.lvclass"> refnum ("Test Pressure.lvclass"), "ReadILCStrategy"=refnum<class "ReadILCDCAPressure3Strategy.lvclass"> refnum ("ReadILCDCAPressure3Strategy.lvclass"), "ConfigureILCStrategy"=refnum<class "ConfigureILCDAC3Strategy.lvclass"> refnum ("ConfigureILCDAC3Strategy.lvclass"), "Pressure Test"=w822, "Sample Delay"=w823, "error in (no error)"=w831, "Test Scenario"=w829, "Log"=w828, "Signal Name"="P3", "Wait"=w824, "Samples To Read"=w825) -> ("Digital Input Test out"=w832:refnum<class "Test Pressure.lvclass">, "error out"=w830:errorcluster)  [unwired: 7 in]
        }
        frame "P3 100%" {
          n135 = Unbundle By Name(w840) -> ("Samples To Average"=w839:i32, "Settling (ms)"=w838:u16, "Delay (ms)"=w837:u16, "100% Test"=w836:T2)
          n136 = call "init.vi"("Digital Input Test in"=refnum<class "Test Pressure.lvclass"> refnum ("Test Pressure.lvclass"), "ReadILCStrategy"=refnum<class "ReadILCDCAPressure3Strategy.lvclass"> refnum ("ReadILCDCAPressure3Strategy.lvclass"), "ConfigureILCStrategy"=refnum<class "ConfigureILCDAC3Strategy.lvclass"> refnum ("ConfigureILCDAC3Strategy.lvclass"), "Pressure Test"=w836, "Sample Delay"=w837, "error in (no error)"=w845, "Test Scenario"=w843, "Log"=w842, "Signal Name"="P3", "Wait"=w838, "Samples To Read"=w839) -> ("Digital Input Test out"=w846:refnum<class "Test Pressure.lvclass">, "error out"=w844:errorcluster)  [unwired: 7 in]
        }
        frame "P4 0%" {
          n137 = Unbundle By Name(w854) -> ("Samples To Average"=w853:i32, "Settling (ms)"=w852:u16, "Delay (ms)"=w851:u16, "0% Test"=w850:T2)
          n138 = call "init.vi"("Digital Input Test in"=refnum<class "Test Pressure.lvclass"> refnum ("Test Pressure.lvclass"), "ReadILCStrategy"=refnum<class "ReadILCDCAPressure4Strategy.lvclass"> refnum ("ReadILCDCAPressure4Strategy.lvclass"), "ConfigureILCStrategy"=refnum<class "ConfigureILCDAC4Strategy.lvclass"> refnum ("ConfigureILCDAC4Strategy.lvclass"), "Pressure Test"=w850, "Sample Delay"=w851, "error in (no error)"=w859, "Test Scenario"=w857, "Log"=w856, "Signal Name"="P4", "Wait"=w852, "Samples To Read"=w853) -> ("Digital Input Test out"=w860:refnum<class "Test Pressure.lvclass">, "error out"=w858:errorcluster)  [unwired: 7 in]
        }
        frame "P4 25%" {
          n139 = Unbundle By Name(w868) -> ("Samples To Average"=w867:i32, "Settling (ms)"=w866:u16, "Delay (ms)"=w865:u16, "25% Test"=w864:T2)
          n140 = call "init.vi"("Digital Input Test in"=refnum<class "Test Pressure.lvclass"> refnum ("Test Pressure.lvclass"), "ReadILCStrategy"=refnum<class "ReadILCDCAPressure4Strategy.lvclass"> refnum ("ReadILCDCAPressure4Strategy.lvclass"), "ConfigureILCStrategy"=refnum<class "ConfigureILCDAC4Strategy.lvclass"> refnum ("ConfigureILCDAC4Strategy.lvclass"), "Pressure Test"=w864, "Sample Delay"=w865, "error in (no error)"=w873, "Test Scenario"=w871, "Log"=w870, "Signal Name"="P4", "Wait"=w866, "Samples To Read"=w867) -> ("Digital Input Test out"=w874:refnum<class "Test Pressure.lvclass">, "error out"=w872:errorcluster)  [unwired: 7 in]
        }
        frame "P4 50%" {
          n141 = Unbundle By Name(w882) -> ("Samples To Average"=w881:i32, "Settling (ms)"=w880:u16, "Delay (ms)"=w879:u16, "50% Test"=w878:T2)
          n142 = call "init.vi"("Digital Input Test in"=refnum<class "Test Pressure.lvclass"> refnum ("Test Pressure.lvclass"), "ReadILCStrategy"=refnum<class "ReadILCDCAPressure4Strategy.lvclass"> refnum ("ReadILCDCAPressure4Strategy.lvclass"), "ConfigureILCStrategy"=refnum<class "ConfigureILCDAC4Strategy.lvclass"> refnum ("ConfigureILCDAC4Strategy.lvclass"), "Pressure Test"=w878, "Sample Delay"=w879, "error in (no error)"=w887, "Test Scenario"=w885, "Log"=w884, "Signal Name"="P4", "Wait"=w880, "Samples To Read"=w881) -> ("Digital Input Test out"=w888:refnum<class "Test Pressure.lvclass">, "error out"=w886:errorcluster)  [unwired: 7 in]
        }
        frame "P4 75%" {
          n143 = Unbundle By Name(w896) -> ("Samples To Average"=w895:i32, "Settling (ms)"=w894:u16, "Delay (ms)"=w893:u16, "75% Test"=w892:T2)
          n144 = call "init.vi"("Digital Input Test in"=refnum<class "Test Pressure.lvclass"> refnum ("Test Pressure.lvclass"), "ReadILCStrategy"=refnum<class "ReadILCDCAPressure4Strategy.lvclass"> refnum ("ReadILCDCAPressure4Strategy.lvclass"), "ConfigureILCStrategy"=refnum<class "ConfigureILCDAC4Strategy.lvclass"> refnum ("ConfigureILCDAC4Strategy.lvclass"), "Pressure Test"=w892, "Sample Delay"=w893, "error in (no error)"=w901, "Test Scenario"=w899, "Log"=w898, "Signal Name"="P4", "Wait"=w894, "Samples To Read"=w895) -> ("Digital Input Test out"=w902:refnum<class "Test Pressure.lvclass">, "error out"=w900:errorcluster)  [unwired: 7 in]
        }
        frame "P4 100%" {
          n145 = Unbundle By Name(w910) -> ("Samples To Average"=w909:i32, "Settling (ms)"=w908:u16, "Delay (ms)"=w907:u16, "100% Test"=w906:T2)
          n146 = call "init.vi"("Digital Input Test in"=refnum<class "Test Pressure.lvclass"> refnum ("Test Pressure.lvclass"), "ReadILCStrategy"=refnum<class "ReadILCDCAPressure4Strategy.lvclass"> refnum ("ReadILCDCAPressure4Strategy.lvclass"), "ConfigureILCStrategy"=refnum<class "ConfigureILCDAC4Strategy.lvclass"> refnum ("ConfigureILCDAC4Strategy.lvclass"), "Pressure Test"=w906, "Sample Delay"=w907, "error in (no error)"=w915, "Test Scenario"=w913, "Log"=w912, "Signal Name"="P4", "Wait"=w908, "Samples To Read"=w909) -> ("Digital Input Test out"=w916:refnum<class "Test Pressure.lvclass">, "error out"=w914:errorcluster)  [unwired: 7 in]
        }
        frame "DCA 1 Linearity" {
          n147 = Unbundle By Name(w918) -> ("Linearity Step"=w919:i32, "DAQ Channel 1 to Read"=w923:refnum<k21>, "DAQ Channel 2 to Read"=w922:refnum<k21>, "Resistor Ohms"=w924:dbl, "Samples To Average"=w925:i32)
          n148 = call "init.vi"("Constant Analog Output Voltage Test in"=refnum<class "Current Linear Test.lvclass"> refnum ("Current Linear Test.lvclass"), "DAQ Channel 1"=w923, "ConfigureILCStrategy"=refnum<class "ConfigureILCDCADAC1Strategy.lvclass"> refnum ("ConfigureILCDCADAC1Strategy.lvclass"), "Counts Per Iteration"=w919, "Samples To Average"=w925, "error in (no error)"=w929, "DAQ Channel 2"=w922, "Log"=w926, "Test Scenario"=w928, "Resistance"=w924, "Signal Name"="DCA 1") -> ("Constant Analog Output Voltage Test  out"=w930:refnum<class "Current Linear Test.lvclass">, "error out"=w927:errorcluster)  [unwired: 7 in]
        }
        frame "DCA 2 Linearity" {
          n149 = Unbundle By Name(w933) -> ("Linearity Step"=w934:i32, "DAQ Channel 1 to Read"=w937:refnum<k21>, "DAQ Channel 2 to Read"=w936:refnum<k21>, "Resistor Ohms"=w938:dbl, "Samples To Average"=w939:i32)
          n150 = call "init.vi"("Constant Analog Output Voltage Test in"=refnum<class "Current Linear Test.lvclass"> refnum ("Current Linear Test.lvclass"), "DAQ Channel 1"=w937, "ConfigureILCStrategy"=refnum<class "ConfigureILCDCADAC2Strategy.lvclass"> refnum ("ConfigureILCDCADAC2Strategy.lvclass"), "Counts Per Iteration"=w934, "Samples To Average"=w939, "error in (no error)"=w943, "DAQ Channel 2"=w936, "Log"=w940, "Test Scenario"=w942, "Resistance"=w938, "Signal Name"="DCA 2") -> ("Constant Analog Output Voltage Test  out"=w944:refnum<class "Current Linear Test.lvclass">, "error out"=w941:errorcluster)  [unwired: 7 in]
        }
      }
    }
    frame Error {
    }
  }
  "error out" <- w3
  "TestScenarioFactory out" <- w5
  "ITestScenario.lvclass" <- w1
